vi "hostCommander.vi"() -> ()   [LabVIEW 2014]
uses:
  <vilib>/Platform/TimedLoop/XDataNode/timing_clust.ctl
  <vilib>/Platform/TimedLoop/XDataNode/nitl_modes.ctl
  <vilib>/Platform/TimedLoop/XDataNode/wakeup.ctl
  <vilib>/dex/Stream Element Allocation Mode.ctl
  <vilib>/platform/TimedLoop/XDataNode/XDataNode.xnode
  <resource>/objmgr/ni.dex.rc
  <vilib>/Platform/TimedLoop/XDataNode/XDNodeRunTimeDep.lvlib
  <vilib>/Analysis/NI_AALBase.lvlib
  <vilib>/Analysis/1siggen.llb/Riffle Array (I32).vi
panel:
  in  "Path":path
  in  "allowCorrection 2":bool
  out "Tab Control":enum32{"Host Commander"}(tab)
  out "rightReward":dbl format="%.2f"
  out "leftReward":dbl format="%.2f"
  out "rightLick":dbl format="%.2f"
  out "leftLick":dbl format="%.2f"
  out "reward#":i32=500
  in  "tickRate":u32=1
  in  "displayLength":dbl=10.0
  out "CurTrial#":u16
  out "Digital Waveform Graph":digitalwaveform(graph)
  out "stateMissed":bool
  out "VSmissed":bool
  out "VSbusy":bool=TRUE caption="VS"
  out "stateBusy":bool=TRUE caption="State"
  in  "FileName":string="debug"
  in  "Save data":bool=TRUE
  in  "Tab Control _2":T1(tab)
  in  "trialKey":i32[](array[numeric])
  in  "left":dbl=0.5 format="%.2f"
  in  "right":dbl=0.5 format="%.2f"
  in  "Initializeation Screen":dbl
  in  "Repeat":dbl
  in  "Interleave":bool
  in  "Randominze":bool
  in  "Blank":bool
  in  "Timing":sgl[](array[numeric])=[0.1, 0.2, 0.4, 0.6, 0.8, 1.0]
  in  "Orientation":sgl[](array[numeric])=[0.1, 0.2, 0.4, 0.6, 0.8, 1.0]
  in  "TF":sgl[](array[numeric])=[0.1, 0.2, 0.4, 0.6, 0.8, 1.0]
  in  "VS type":string="LR_FullFiledGrating"
  in  "SF":sgl[](array[numeric])=[0.04, 0.08, 0.16, 0.32, 0.45]
  in  "rtFIFOsize":u32=50
  in  "rtFIFOtimeout":u32
  in  "rtFIFOdataPool":u32=20
  in  "stateMachineCycle_uS":i64=500
  in  "minDelay":i32=2000000
  in  "maxDelay":i32=2000000
  in  "autoAllowCorrection":bool
  in  "allowCorrection":bool
  in  "autoDelay":bool
  in  "vsFilterPeriod_uS":i32=500 format="%#1.6f"
  in  "lickThreshold_V":fxp<+/-,16,5>=1.0 format="%#.4f"
  in  "vsThreshold_V":fxp<+/-,16,5>=2.0 format="%#.4f"
  in  "audioThreshold_V":fxp<+/-,16,5>=2.2998046875 format="%.4f"
  in  "audioFilterPeriod_uS":i32=500 format="%#1.6f"
  in  "audioOffState_V":fxp<+/-,16,5> format="%#.4f"
  in  "manualShock":bool
  in  "manualWaterRight":bool
  in  "manualWaterLeft":bool
  in  "lickReward":bool
  in  "allowPunish":bool
  in  "beh type":string="LeftRight"
  in  "toneReward":bool
  in  "rwdrefPeriod_uS":u32=1000000
  in  "rewardPeriod_uS":u32=3000000
  in  "waterOn_uS":u32=35000
  in  "timeout_uS":u32
  in  "shockOn_uS":u32
  in  "delay_uS":u32
  out "current state":u16(ring) items=["idle", "vs before", "vs", "vs after", "delay", "tone before", "tone", "tone after", "cycle end", "reward", "reward refractory", "punish", "punish refractory", "timeout", "exit"]
  out "case2":i32
  out "case1":i32
  in  "forceLeftTrial":bool
  in  "forceRightTrial":bool
  in  "forceCorrTrial":bool
  in  "autoCorrTrial":bool
  in  "autoTimeout":bool
  in  "autoStop":bool
  in  "autoStopAtReward#":i32=250
  in  "updateEveryTrial#":u16=10
  in  "maxTimeout":i32=8000000
  out "newStartTrial#":i32
  out "newStartReward#":i32
  out "contNoRewardAccum":i32
  out "contNoReward":i32
  out "contReward":i32
  out "curPerformance":dbl format="%.2f"
  out "overallPerformance":dbl format="%.2f"
  in  "waterPunish":bool
  out "Error 1":string
  out "Error 2":string
  out "Originating IP":string="192.168.137.2"
  out "Incoming data":string="TrlDone 1.000 "
  out "stream counter":u32
  out "Is Connected":bool
  out "Available Elements for Writing":i32
  in  "stream writer buffer size":i32=500
  in  "IP_VS":string="192.168.137.3"
  in  "IP_RT":string="192.168.137.2"
  in  "port_remote":u16=9091
  in  "IP_host":string="192.168.137.1"
  in  "port_local":u16=9090
  in  "IP_broadcast":string="192.168.137.255"
  out "INFO":string="Stop 1.000 "
  out "stop - local":bool=TRUE
  in  "Notes":string="14-4"
  in  "Abort":bool caption="run-stop"
  in  "run-stop":bool
  out "dispTimeout":bool
  out "saveTimeout":bool
  out "CurTrial# (remote)":u16
  in  "totalTrial#":u16=600
  out "CurTime":i32
  in  "ITI_ms":dbl=2000.0
  out "CurTime (sec)":i32
  in  "FilePath":string="D:\\BehData\\"
  # "busy"
  # "missed"
  # "min"
  # "sec"
  # "trialProbability"
  # "Errors for debugging"
types:
  T1 = enum32{"Visual Stimuli", "State Machine", "Behavior", "Network", "Notes"}
  T2 = enum16{"open", "replace", "create", "open or create", "replace or create", "replace or create with confirmation"}
  T3 = enum16{"big-endian, network order", "native, host order", "little-endian"}
  T4 = typedef "XDNodeRunTimeDep.lvlib/timing_clust.ctl" = cluster{"Expected End [f-1]":u64, "Actual End [f-1]":u64, "Finished Late? [f-1]":bool, "Expected End [i-1]":u64, "Actual End [i-1]":u64, "Finished Late? [i-1]":bool, "Expected Start [i]":u64, "Actual Start [i]":u64, "Expected Start [f]":u64, "Actual Start [f]":u64, "Source Name":string, "Structure Name":string, "Period":i64, "Deadline":i64, "Offset":i64, "Start":i64, "Priority":i32, "Timeout":i32, "Mode":T5, "Wakeup Reason":T6, "Error":errorcluster, "Source Type":string, "Secondary Source Type":string, "Global End Time":u64, "Global Start Time":u64, "Frame Duration":u64, "Iteration Duration":u64, "Assigned CPU":i32, "I/O Scan Engine Mode":u32}
  T5 = typedef "XDNodeRunTimeDep.lvlib/nitl_modes.ctl" = enum32{"No Change", "Process missed periods, maintain original phase", "Discard missed periods, maintain original phase", "Process missed periods, ignore original phase", "Discard missed periods, ignore original phase"}
  T6 = typedef "XDNodeRunTimeDep.lvlib/wakeup.ctl" = enum32{"Normal", "Aborted", "Asynchronous wakeup", "Timing source error", "Timed loop error", "Timeout"}
  T7 = typedef "Stream Element Allocation Mode.ctl" = u32
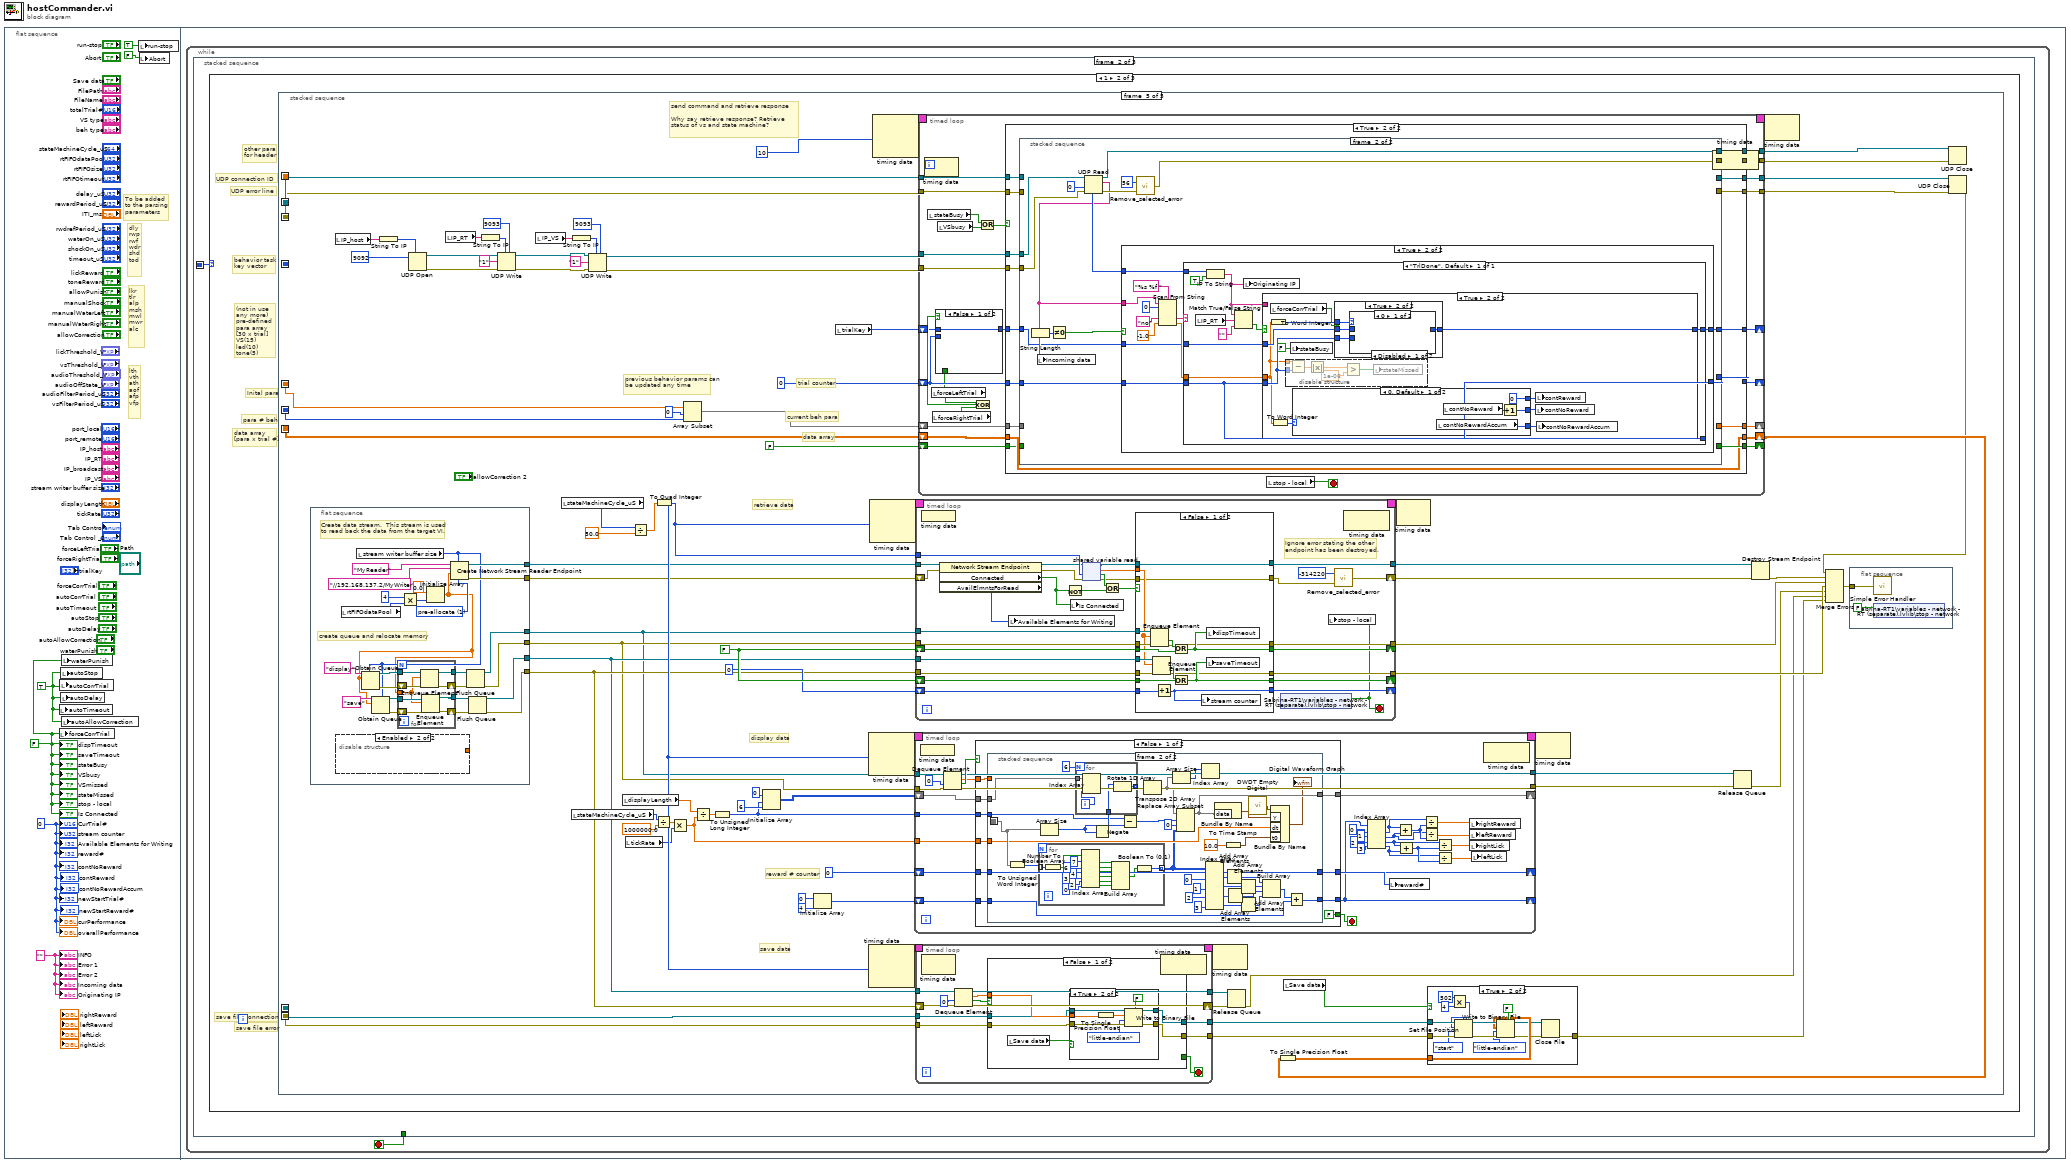
[diagram p0: block diagram]
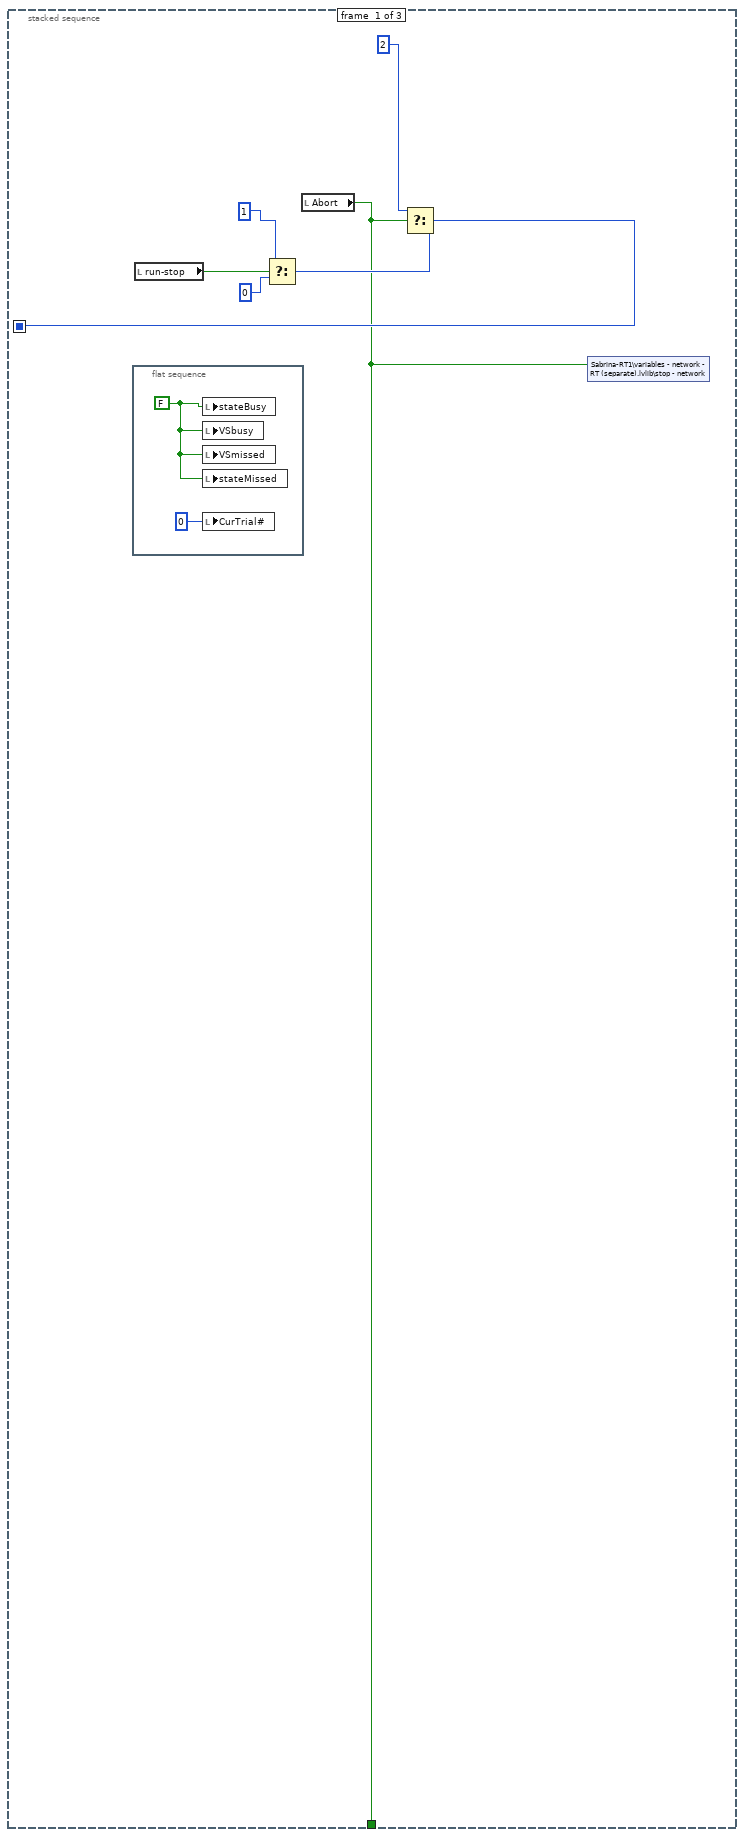
[diagram p2: hidden frame]
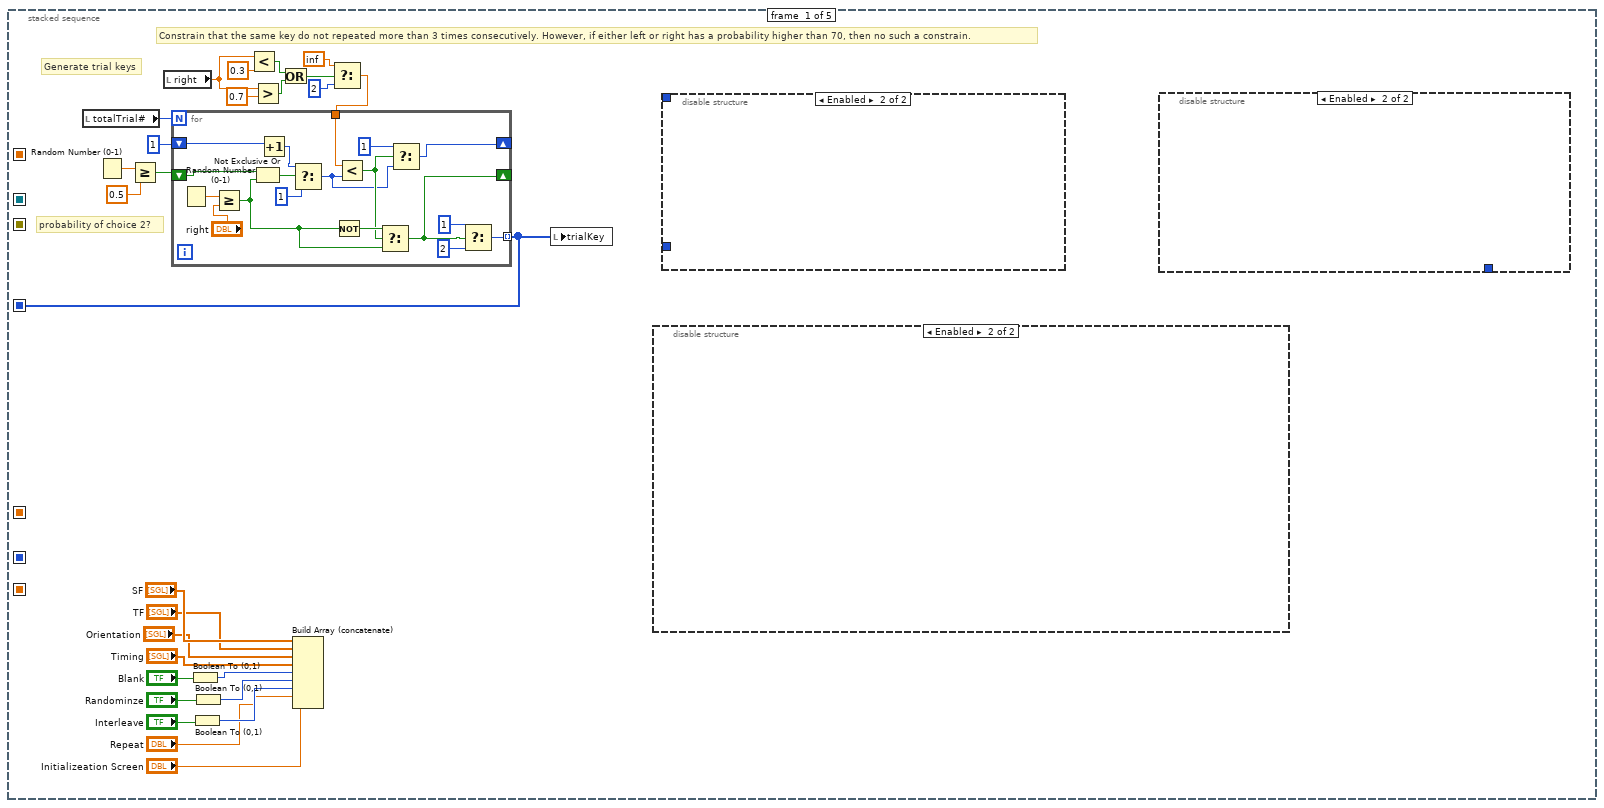
[diagram p4: hidden frame]
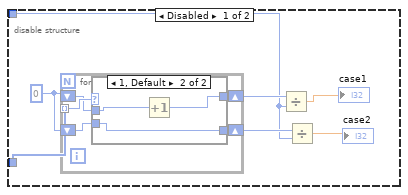
[diagram p5: hidden frame]
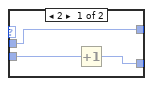
[diagram p6: hidden frame]
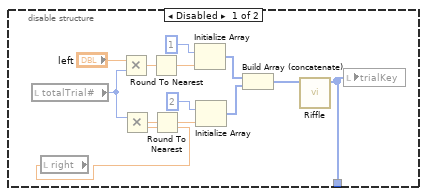
[diagram p7: hidden frame]
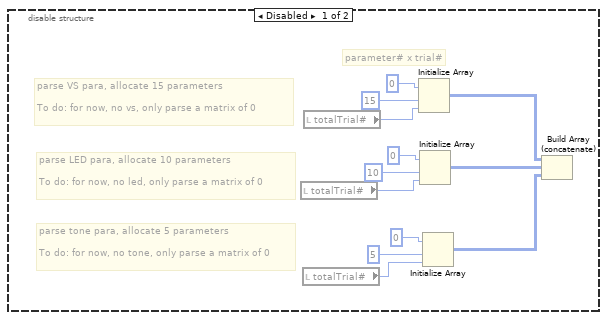
[diagram p8: hidden frame]
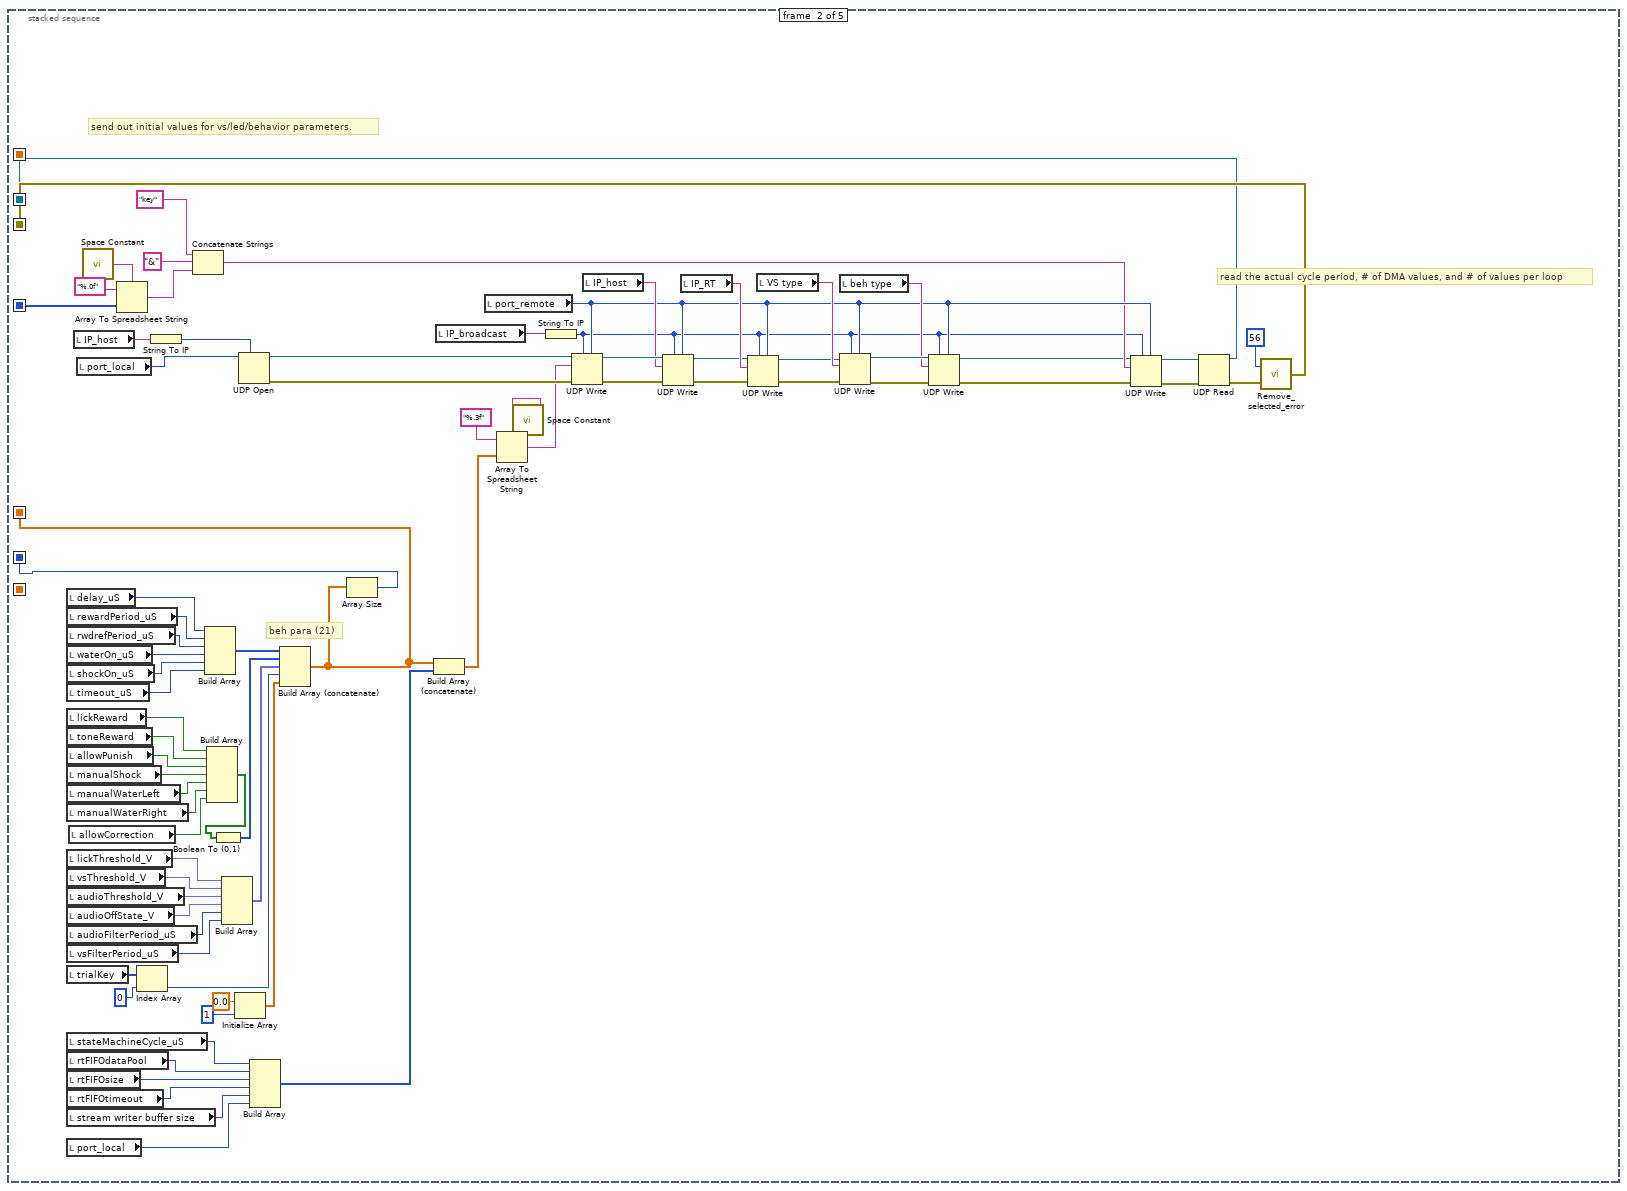
[diagram p9: hidden frame]
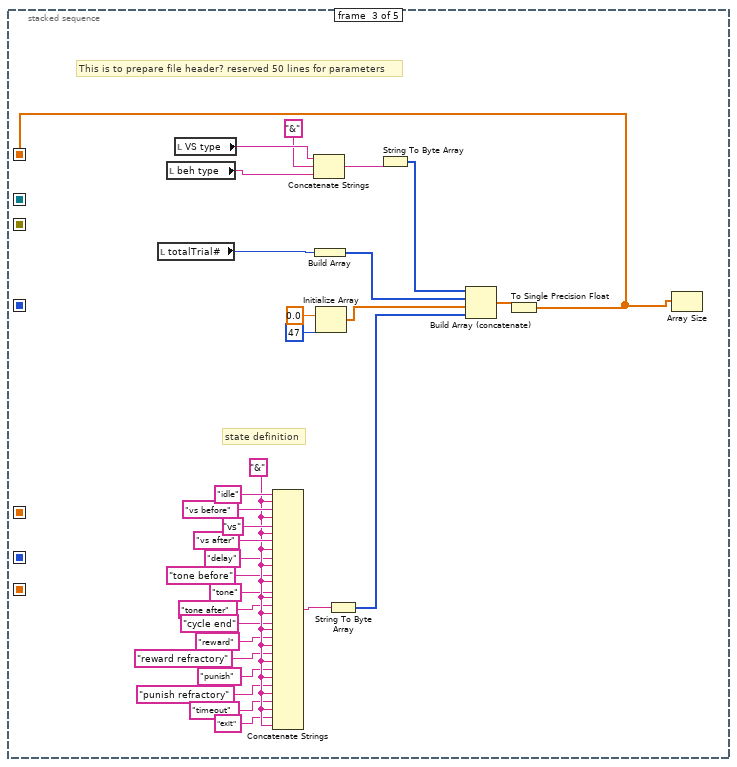
[diagram p10: hidden frame]
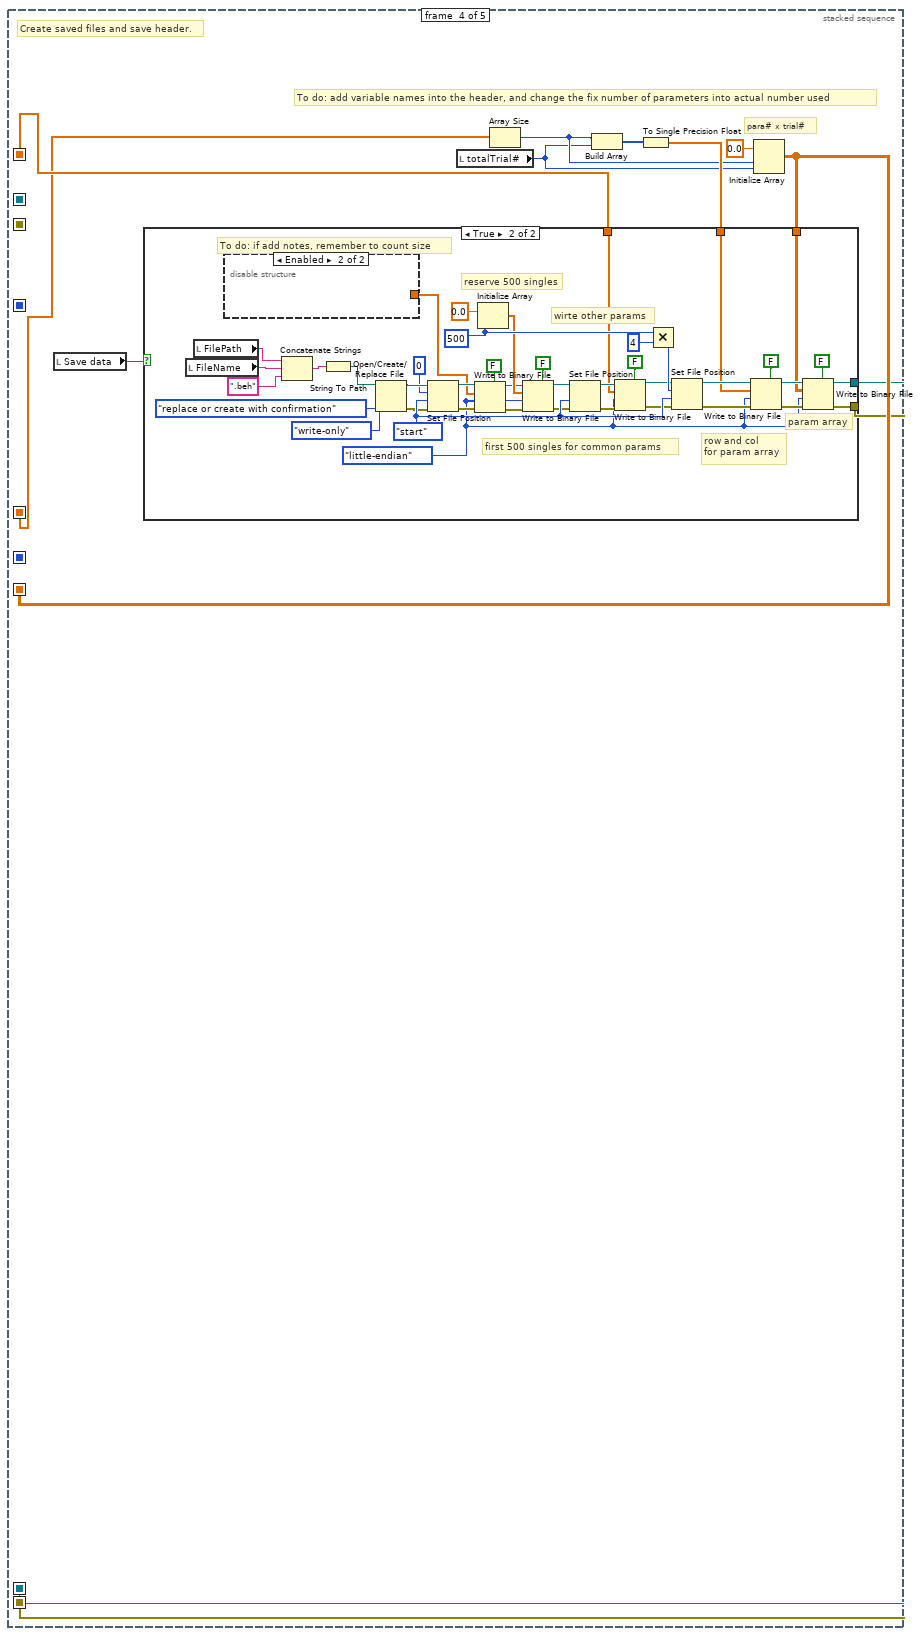
[diagram p11: hidden frame]
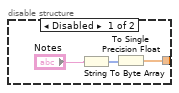
[diagram p13: hidden frame]
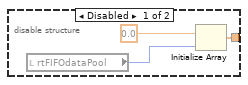
[diagram p14: hidden frame]
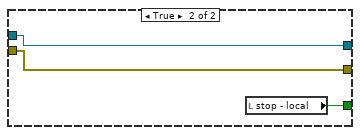
[diagram p16: hidden frame]
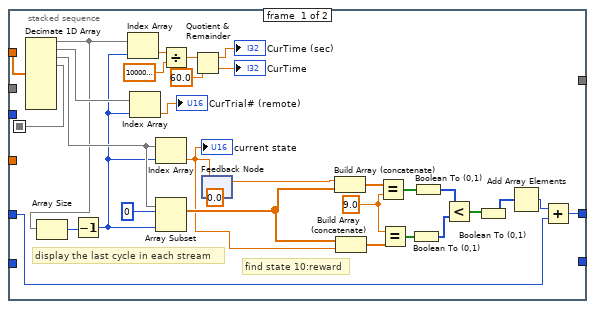
[diagram p17: hidden frame]
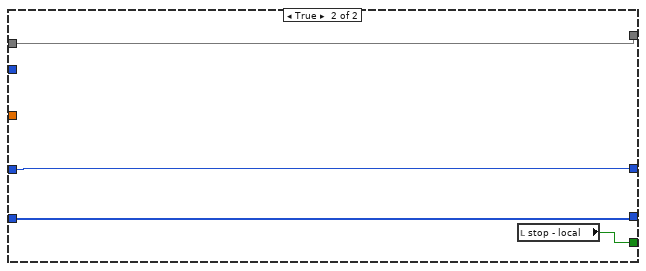
[diagram p18: hidden frame]
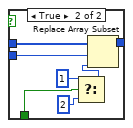
[diagram p20: hidden frame]
diagram:
  n1 = flat-sequence {
    frame #0 {
      w2 = TRUE
      w4 = ""
      w3 = 0
      w1 = FALSE
      # "To be added\nto the parsing\nparameters"
      # "lth\nvth\nath\naof\nafp\nvfp"
      # "dly\nrwp\nrwf\nwdr\nshd\ntod"
      # "lkr\ntlr\nalp\nmsh\nmwl\nmwr\nalc"
      n2 = local write "autoTimeout"(w2) -> ()
      n3 = local write "forceCorrTrial"(w1) -> ()
      n4 = local write "autoCorrTrial"(w2) -> ()
      n5 = local write "autoDelay"(w2) -> ()
      n6 = local write "autoStop"(w2) -> ()
      n7 = local write "waterPunish"(w1) -> ()
      n8 = local write "autoAllowCorrection"(w2) -> ()
      n9 = local write "run-stop"(TRUE) -> ()
      n10 = local write "Abort"(FALSE) -> ()
      "dispTimeout" <- w1
      "saveTimeout" <- w1
      "stateBusy" <- w1
      "VSbusy" <- w1
      "VSmissed" <- w1
      "stateMissed" <- w1
      "CurTrial#" <- w3
      "stop - local" <- w1
      "INFO" <- w4
      "Error 2" <- w4
      "Error 1" <- w4
      "Available Elements for Writing" <- w3
      "Is Connected" <- w1
      "stream counter" <- w3
      "Incoming data" <- w4
      "Originating IP" <- w4
      "reward#" <- w3
      "contNoReward" <- w3
      "contReward" <- w3
      "contNoRewardAccum" <- w3
      "newStartTrial#" <- w3
      "newStartReward#" <- w3
      "curPerformance" <- w3
      "overallPerformance" <- w3
    }
    frame #1 {
      n11 = while {
        stop <- w7 stop-if-true
        n12 = stacked-sequence {
          seq-local: [w9 _ _] -> [_ w17 _]
          tunnel: [w8 _ _] -> w7
          frame #0 {
            n13 = flat-sequence {
              frame #0 {
                w16 = FALSE
                n14 = local write "stateBusy"(w16) -> ()
                n15 = local write "VSbusy"(w16) -> ()
                n16 = local write "VSmissed"(w16) -> ()
                n17 = local write "stateMissed"(w16) -> ()
                n18 = local write "CurTrial#"(0) -> ()
              }
            }
            n19 = local read "run-stop"() -> (w11:bool)
            n20 = Select(t=u8 1, s=w11, f=u8 0) -> (s? t:f=w10:u8)
            n21 = local read "Abort"() -> (w8:bool)
            n22 = Select(t=u8 2, s=w8, f=w10) -> (s? t:f=w9:u8)
            n23 = shared-variable "Sabrina-RT1\\variables - network - RT (separate).lvlib\\stop - network"(w8) -> ()  [unwired: 1 in, 1 out]
          }
          frame #1 {
            n24 = case shown="1" w17 {
              frame 0, Default {
              }
              frame 1 {
                # "behavior task\nkey vector"
                # "para # beh"
                # "save file error"
                # "save file connection"
                # "data array\n[para x trial #]"
                # "other para\nfor header"
                # "UDP error line"
                # "UDP connection ID"
                # "Inital para"
                # "(not in use any more) pre-defined \npara array\n[30 x trial]\nVS(15)\nled(10)\ntone(5)"
                n25 = stacked-sequence {
                  seq-local: [_ w166 _ _ _] -> [_ _ _ _ w342]
                  seq-local: [_ w165 _ _ _] -> [_ _ _ _ w343]
                  seq-local: [_ w125 _ _ _] -> [_ _ _ w215 w291]
                  seq-local: [w18 _ _ _ _] -> [_ w121 _ _ _]
                  seq-local: [_ _ w183 _ _] -> [_ _ _ w219 _]
                  seq-local: [_ _ _ w218 _] -> [_ _ _ _ w336]
                  seq-local: [_ _ _ w217 _] -> [_ _ _ _ w316]
                  seq-local: [_ _ _ w216 _] -> [_ _ _ _ w317]
                  seq-local: [_ w134 _ _ _] -> [_ _ _ _ w297]
                  frame #0 {
                    # "probability of choice 2?"
                    # "Constrain that the same key do not repeated more than 3 times consecutively. However, if either left or right has a probability higher than 70, then no such a constrain."
                    # "Generate trial keys"
                    n26 = local read "totalTrial#"() -> (w19:u16)
                    n27 = Random Number (0-1)() -> (number: 0 to 1=w32:dbl)
                    n28 = Greater Or Equal?(x=w32, y=0.5) -> (x >= y?=w30:bool)
                    n29 = local read "right"() -> (w26:dbl)
                    n30 = Boolean To (0,1)(Boolean="Blank") -> (0, 1=w39:i16)
                    n31 = Boolean To (0,1)(Boolean="Interleave") -> (0, 1=w34:i16)
                    n32 = Boolean To (0,1)(Boolean="Randominze") -> (0, 1=w38:i16)
                    n33 = Less?(x=w26, y=0.3) -> (x < y?=w23:bool)
                    n34 = Greater?(x=w26, y=0.7) -> (0:w22:bool)
                    n35 = Or(x=w23, y=w22) -> (x .or. y?=w21:bool)
                    n36 = Build Array (concatenate)("SF", "TF", "Orientation", "Timing", w39, w38, w34, "Repeat", "Initializeation Screen") -> ()  [unwired: 1 out]
                    n37 = Select(t=inf, s=w21, f=2) -> (s? t:f=w20:dbl)
                    n38 = for {
                      N: w19 -> [_]
                      shift-right: [w79] -> _
                      shift-left: w30 -> [w92]
                      shift-right: [w77] -> _
                      shift-left: 1 -> [w90]
                      tunnel: w20 -> [w80]
                      tunnel: [w78] -> w18 mode=indexing
                      n39 = Random Number (0-1)() -> (number: 0 to 1=w93:dbl)
                      n40 = Greater Or Equal?(x=w93, y="right") -> (x >= y?=w83:bool)
                      n41 = Not Exclusive Or(1:w83, 2:w92) -> (0:w91:bool)
                      n42 = Increment(x=w90) -> (x+1=w87:i32)
                      n43 = Select(t=w87, s=w91, f=1) -> (s? t:f=w81:i32)
                      n44 = Not(x=w83) -> (.not. x?=w84:bool)
                      n45 = Less?(x=w80, y=w81) -> (x < y?=w82:bool)
                      n46 = Select(t=w84, s=w82, f=w83) -> (s? t:f=w79:bool)
                      n47 = Select(t=1, s=w82, f=w81) -> (s? t:f=w77:i32)
                      n48 = Select(t=1, s=w79, f=2) -> (s? t:f=w78:i32)
                    }
                    n49 = local write "trialKey"(w18) -> ()
                    n50 = disable-structure shown="Enabled" {
                      frame Disabled {
                        # "parameter# x trial#"
                        # "parse tone para, allocate 5 parameters \n\nTo do: for now, no tone, only parse a matrix of 0"
                        # "parse LED para, allocate 10 parameters \n\nTo do: for now, no led, only parse a matrix of 0"
                        # "parse VS para, allocate 15 parameters \n\nTo do: for now, no vs, only parse a matrix of 0"
                        n51 = local read "totalTrial#"() -> (w99:u16)
                        n52 = local read "totalTrial#"() -> (w98:u16)
                        n53 = local read "totalTrial#"() -> (w100:u16)
                        n54 = Initialize Array(0, 15, w100) -> (w103:i32[][])
                        n55 = Initialize Array(0, 10, w99) -> (w102:i32[][])
                        n56 = Initialize Array(0, 5, w98) -> (w101:i32[][])
                        n57 = Build Array (concatenate)(w103, w102, w101) -> ()  [unwired: 1 out]
                      }
                      frame Enabled {
                      }
                    }
                    n58 = disable-structure shown="Enabled" {
                      disable-tunnel: _ -> [w51 _]
                      disable-tunnel: _ -> [w45 _]
                      frame Disabled {
                        w50 = 0
                        n59 = for {
                          tunnel: w51 -> [w56] mode=indexing
                          shift-right: [w54] -> w47
                          shift-left: w50 -> [w55]
                          shift-right: [w52] -> w49
                          shift-left: w50 -> [w53]
                          n60 = case shown="1, Default" w56 {
                            tunnel: w55 -> [w59 w60]
                            tunnel: [w58 w60] -> w54
                            tunnel: w53 -> [w57 w62]
                            tunnel: [w57 w61] -> w52
                            frame 2 {
                              n61 = Increment(x=w59) -> (x+1=w58:i32)
                            }
                            frame 1, Default {
                              n62 = Increment(x=w62) -> (x+1=w61:i32)
                            }
                          }
                        }
                        n63 = Divide(x=w49, y=w45) -> (x/y=→"case1":dbl)
                        n64 = Divide(x=w47, y=w45) -> (x/y=→"case2":dbl)
                      }
                      frame Enabled {
                      }
                    }
                    n65 = disable-structure shown="Enabled" {
                      disable-tunnel: [w64 _] -> _
                      frame Disabled {
                        n66 = local read "totalTrial#"() -> (w68:u16)
                        n67 = local read "right"() -> (w63:dbl)
                        n68 = Multiply(x="left", y=w68) -> (x*y=w74:dbl)
                        n69 = Multiply(x=w68, y=w63) -> (x*y=w69:dbl)
                        n70 = Round To Nearest(number=w74) -> (nearest integer value=w72:dbl)
                        n71 = Round To Nearest(number=w69) -> (nearest integer value=w71:dbl)
                        n72 = Initialize Array(1, w72) -> (w67:i32[])
                        n73 = Initialize Array(2, w71) -> (w66:i32[])
                        n74 = Build Array (concatenate)(w67, w66) -> (w65:i32[])
                        n75 = call-poly <vilib>:"Riffle.vi"("X"=w65) -> ("Riffled {X}"=w64:i32[])  [unwired: 8 in, 2 out]
                        n76 = local write "trialKey"(w64) -> ()
                      }
                      frame Enabled {
                      }
                    }
                  }
                  frame #1 {
                    # "beh para (21)"
                    # "read the actual cycle period, # of DMA values, and # of values per loop"
                    # "send out initial values for vs/led/behavior parameters."
                    n77 = local read "delay_uS"() -> (w162:u32)
                    n78 = local read "rewardPeriod_uS"() -> (w161:u32)
                    n79 = local read "rwdrefPeriod_uS"() -> (w160:u32)
                    n80 = local read "waterOn_uS"() -> (w159:u32)
                    n81 = local read "shockOn_uS"() -> (w158:u32)
                    n82 = local read "timeout_uS"() -> (w157:u32)
                    n83 = local read "lickReward"() -> (w156:bool)
                    n84 = local read "toneReward"() -> (w155:bool)
                    n85 = local read "allowPunish"() -> (w154:bool)
                    n86 = local read "manualShock"() -> (w153:bool)
                    n87 = local read "manualWaterLeft"() -> (w152:bool)
                    n88 = local read "manualWaterRight"() -> (w151:bool)
                    n89 = local read "lickThreshold_V"() -> (w150:fxp<+/-,16,5>)
                    n90 = local read "vsThreshold_V"() -> (w149:fxp<+/-,16,5>)
                    n91 = local read "audioThreshold_V"() -> (w148:fxp<+/-,16,5>)
                    n92 = local read "audioOffState_V"() -> (w145:fxp<+/-,16,5>)
                    n93 = local read "audioFilterPeriod_uS"() -> (w147:i32)
                    n94 = local read "vsFilterPeriod_uS"() -> (w146:i32)
                    n95 = local read "trialKey"() -> (w110:i32[])
                    n96 = local read "stateMachineCycle_uS"() -> (w144:i64)
                    n97 = local read "rtFIFOdataPool"() -> (w142:u32)
                    n98 = local read "rtFIFOsize"() -> (w141:u32)
                    n99 = local read "rtFIFOtimeout"() -> (w143:u32)
                    n100 = local read "stream writer buffer size"() -> (w140:i32)
                    n101 = local read "port_local"() -> (w133:u16)
                    n102 = local read "allowCorrection"() -> (w106:bool)
                    n103 = local read "IP_host"() -> (w179:string)
                    n104 = local read "port_local"() -> (w178:u16)
                    n105 = call <vilib>:"Space Constant.vi"() -> ("String"=w115:string)
                    n106 = Array To Spreadsheet String ("beh para")(delimiter (Tab)=w115, array=w121, 3:"%.0f" ("format string")) -> (spreadsheet string=w117:string)
                    n107 = Index Array(array=w110, index=0) -> (element=w107:i32)
                    n108 = String To IP(1:w179) -> (0:w111:u32)
                    n109 = Concatenate Strings("key", "&", w117) -> (w116:string)
                    n110 = Build Array(w162, w161, w160, w159, w158, w157) -> (w139:u32[])
                    n111 = Build Array(w156, w155, w154, w153, w152, w151, w106) -> (w127:bool[])
                    n112 = Boolean To (0,1)(Boolean=w127) -> (0, 1=w126:i16[])
                    n113 = Build Array(w150, w149, w148, w145, w147, w146) -> (w138:fxp<+/-,43,32>[])
                    n114 = Initialize Array(sgl 0.0, 1) -> (w108:sgl[])
                    n115 = UDP Open(7:w111, 11:w178) -> (port=w176:refnum<k16>, 0:w177:errorcluster)  [unwired: 3 in, 1 out]
                    n116 = Build Array(w144, w142, w141, w143, w140, w133) -> (w137:i64[])
                    n117 = Build Array (concatenate)(w139, w126, w138, w107, w108) -> (w125:sgl[])
                    n118 = Array Size(array=w125) -> (size(s)=w134:i32)
                    n119 = Build Array (concatenate)(w125, w137) -> (w167:sgl[])
                    n120 = local read "IP_broadcast"() -> (w180:string)
                    n121 = local read "port_remote"() -> (w118:u16)
                    n122 = call <vilib>:"Space Constant.vi"() -> ("String"=w169:string)
                    n123 = Array To Spreadsheet String ("beh para")(delimiter (Tab)=w169, array=w167, 3:"%.3f" ("format string")) -> (spreadsheet string=w168:string)
                    n124 = String To IP(1:w180) -> (0:w112:u32)
                    n125 = UDP Write(address=w112, port or service name=w118, connection ID=w176, data in=w168, 8:w177) -> (error out=w175:errorcluster, 3:w132:refnum<k16>)  [unwired: 1 in]
                    n126 = local read "IP_host"() -> (w131:string)
                    n127 = UDP Write(address=w112, port or service name=w118, connection ID=w132, data in=w131) -> (3:w129:refnum<k16>)  [unwired: 2 in, 1 out]
                    n128 = local read "IP_RT"() -> (w130:string)
                    n129 = UDP Write(address=w112, port or service name=w118, connection ID=w129, data in=w130) -> (3:w128:refnum<k16>)  [unwired: 2 in, 1 out]
                    n130 = local read "VS type"() -> (w174:string)
                    n131 = local read "beh type"() -> (w171:string)
                    n132 = UDP Write(address=w112, port or service name=w118, connection ID=w128, data in=w174, 8:w175) -> (error out=w173:errorcluster, 3:w172:refnum<k16>)  [unwired: 1 in]
                    n133 = UDP Write(address=w112, port or service name=w118, connection ID=w172, data in=w171, 8:w173) -> (error out=w113:errorcluster, 3:w114:refnum<k16>)  [unwired: 1 in]
                    n134 = UDP Write(address=w112, port or service name=w118, connection ID=w114, data in=w116, 8:w113) -> (error out=w124:errorcluster, 3:w123:refnum<k16>)  [unwired: 1 in]
                    n135 = UDP Read(connection ID=w123, 8:w124) -> (error out=w164:errorcluster, 3:w165:refnum<k16>)  [unwired: 2 in, 3 out]
                    n136 = call "Remove_selected_error.vi"("error in (no error)"=w164, "errorCode"=56) -> ("error out"=w166:errorcluster)
                  }
                  frame #2 {
                    w195 = "&" ("string")
                    # "state definition"
                    # "This is to prepare file header? reserved 50 lines for parameters"
                    n137 = local read "totalTrial#"() -> (w203:u16)
                    n138 = local read "beh type"() -> (w181:string)
                    n139 = local read "VS type"() -> (w198:string)
                    n140 = Concatenate Strings("idle", w195, "vs before", w195, "vs", w195, "vs after", w195, "delay", w195, "tone before", w195, "tone", w195, "tone after", w195, "cycle end", w195, "reward", w195, "reward refractory", w195, "punish", w195, "punish refractory", w195, "timeout", w195, "exit", w195) -> (w208:string)
                    n141 = Concatenate Strings(w198, "&" ("string"), w181) -> (w197:string)
                    n142 = Build Array(w203) -> (w202:u16[])
                    n143 = Initialize Array(sgl 0.0 ("element"), 47 ("dimension size")) -> (w201:sgl[])
                    n144 = String To Byte Array(string=w208) -> (unsigned byte array=w200:u8[])
                    n145 = String To Byte Array(string=w197) -> (unsigned byte array=w196:u8[])
                    n146 = Build Array (concatenate)(w196, w202, w201, w200) -> (w199:sgl[])
                    n147 = To Single Precision Float(number=w199) -> (single precision float=w183:sgl[])
                    n148 = Array Size(array=w183) -> ()  [unwired: 1 out]
                  }
                  frame #3 {
                    # "To do: add variable names into the header, and change the fix number of parameters into actual number used"
                    # "para# x trial#"
                    # "Create saved files and save header."
                    n149 = local read "Save data"() -> (w221:bool)
                    n150 = local read "totalTrial#"() -> (w211:u16)
                    n151 = Array Size(array=w215) -> (size(s)=w212:i32)
                    n152 = Build Array(w212, w211) -> (w214:i32[])
                    n153 = To Single Precision Float(number=w214) -> (single precision float=w213:sgl[])
                    n154 = Initialize Array(sgl 0.0 ("element"), w212, w211) -> (w218:sgl[][])
                    n155 = case shown="True" w221 {
                      tunnel: w213 -> [_ w238]
                      tunnel: w219 -> [_ w222]
                      tunnel: w218 -> [_ w237]
                      tunnel: [_ w235] -> w216
                      tunnel: [_ w236] -> w217
                      frame False {
                      }
                      frame True {
                        w256 = 500 ("dimension size")
                        w229 = T3."little-endian" ("byte order (0:big-endian, network order)")
                        w257 = enum16{"start", "end", "current"}."start" ("from (0:start)")
                        # "To do: if add notes, remember to count size"
                        # "param array"
                        # "row and col\nfor param array"
                        # "first 500 singles for common params"
                        # "reserve 500 singles"
                        # "wirte other params"
                        n156 = local read "FileName"() -> (w224:string)
                        n157 = local read "FilePath"() -> (w227:string)
                        n158 = disable-structure shown="Enabled" {
                          disable-tunnel: [w264 _] -> w228
                          frame Disabled {
                            n159 = String To Byte Array(string="Notes") -> (unsigned byte array=w265:u8[])
                            n160 = To Single Precision Float(number=w265) -> (single precision float=w264:sgl[])
                          }
                          frame Enabled {
                          }
                        }
                        n161 = Concatenate Strings(w227, w224, ".beh" ("string")) -> (w226:string)
                        n162 = String To Path(string=w226) -> (path=w225:path)
                        n163 = Open/Create/Replace File(file path (use dialog)=w225, operation (0:open)=T2."replace or create with confirmation", access (0:read/write)=enum16{"read/write", "read-only", "write-only"}."write-only") -> (refnum out=w242:refnum<file>, error out=w243:errorcluster)  [unwired: 3 in, 1 out]
                        n164 = Set File Position(offset (in bytes) (0)=i64 0, refnum=w242, from (0:start)=w257, error in=w243) -> (refnum out=w233:refnum<file>, error out=w231:errorcluster)
                        n165 = Write to Binary File(file (use dialog)=w233, data=w228, error in=w231, 5:FALSE ("prepend array or string size? (T)"), 9:w229) -> (refnum out=w232:refnum<file>, error out=w230:errorcluster)  [unwired: 1 in, 1 out]
                        n166 = Initialize Array(sgl 0.0 ("element"), w256) -> (w246:sgl[])
                        n167 = Write to Binary File(file (use dialog)=w232, data=w246, error in=w230, 5:FALSE ("prepend array or string size? (T)"), 9:w229) -> (refnum out=w248:refnum<file>, error out=w249:errorcluster)  [unwired: 1 in, 1 out]
                        n168 = Set File Position(refnum=w248, from (0:start)=w257, error in=w249) -> (refnum out=w250:refnum<file>, error out=w251:errorcluster)  [unwired: 1 in]
                        n169 = Write to Binary File(file (use dialog)=w250, data=w222, error in=w251, 5:FALSE ("prepend array or string size? (T)"), 9:w229) -> (refnum out=w252:refnum<file>, error out=w253:errorcluster)  [unwired: 1 in, 1 out]
                        n170 = Multiply(x=w256, y=4) -> (x*y=w254:i32)
                        n171 = Set File Position(offset (in bytes) (0)=w254, refnum=w252, from (0:start)=w257, error in=w253) -> (refnum out=w259:refnum<file>, error out=w260:errorcluster)
                        n172 = Write to Binary File(file (use dialog)=w259, data=w238, error in=w260, 5:FALSE ("prepend array or string size? (T)"), 9:w229) -> (refnum out=w261:refnum<file>, error out=w262:errorcluster)  [unwired: 1 in, 1 out]
                        n173 = Write to Binary File(file (use dialog)=w261, data=w237, error in=w262, 5:FALSE ("prepend array or string size? (T)"), 9:w229) -> (refnum out=w235:refnum<file>, error out=w236:errorcluster)  [unwired: 1 in, 1 out]
                      }
                    }
                  }
                  frame #4 {
                    w348 = FALSE
                    # "reward # counter"
                    # "save data"
                    # "data array"
                    # "current beh para"
                    # "trial counter"
                    # "previous behavior params can be updated any time"
                    # "display data"
                    # "retrieve data"
                    # "send command and retrieve response\n\nWhy say retrieve response? Retrieve\nstatus of vs and state machine?"
                    n174 = flat-sequence {
                      tunnel: [w375] -> w303
                      tunnel: [w374] -> w302
                      tunnel: [w363] -> w301
                      tunnel: [w362] -> w300
                      tunnel: [w361] -> w299
                      tunnel: [w360] -> w298
                      frame #0 {
                        w377 = T7 1 items=["allocate as needed", "pre-allocate"] ("element allocation mode")
                        # "create queue and relocate memory"
                        # "Create data stream.  This stream is used\nto read back the data from the target VI."
                        n175 = disable-structure shown="Enabled" {
                          disable-tunnel: [w380 _] -> _
                          frame Disabled {
                            n176 = local read "rtFIFOdataPool"() -> (w381:u32)
                            n177 = Initialize Array(sgl 0.0, w381) -> (w380:sgl[])
                          }
                          frame Enabled {
                          }
                        }
                        n178 = local read "rtFIFOdataPool"() -> (w356:u32)
                        n179 = local read "stream writer buffer size"() -> (w359:i32)
                        n180 = Multiply(x=4, y=w356) -> (x*y=w355:u32)
                        n181 = Initialize Array(sgl 0.0, w355) -> (w358:sgl[])
                        n182 = Obtain Queue(max queue size (-1, unlimited)=w359, name (unnamed)="display", element data type=w358) -> (queue out=w366:refnum<queue>, error out=w367:errorcluster)  [unwired: 2 in, 1 out]
                        n183 = Obtain Queue(max queue size (-1, unlimited)=w359, name (unnamed)="save", element data type=w358) -> (queue out=w368:refnum<queue>, error out=w369:errorcluster)  [unwired: 2 in, 1 out]
                        n184 = for {
                          N: w359 -> [_]
                          tunnel: w366 -> [w391]
                          tunnel: [w390] -> w372
                          shift-right: [w388] -> w373
                          shift-left: w367 -> [w389]
                          shift-right: [w384] -> w371
                          shift-left: w369 -> [w385]
                          tunnel: w368 -> [w387]
                          tunnel: [w386] -> w370
                          tunnel: w358 -> [w383]
                          n185 = Enqueue Element(queue=w391, element=w383, error in (no error)=w389) -> (queue out=w390:refnum<queue>, error out=w388:errorcluster)  [unwired: 1 in, 1 out]
                          n186 = Enqueue Element(queue=w387, element=w383, error in (no error)=w385) -> (queue out=w386:refnum<queue>, error out=w384:errorcluster)  [unwired: 1 in, 1 out]
                        }
                        n187 = Create Network Stream Reader Endpoint(6:w377, 7:w359, 9:w358, 10:"//192.168.137.2/MyWriter" ("reader name"), 11:"MyReader" ("reader name")) -> (0:w375:errorcluster, 3:w374:refnum<k21>)  [unwired: 2 in]
                        n188 = Flush Queue(queue=w372, error in (no error)=w373) -> (queue out=w360:refnum<queue>, error out=w361:errorcluster)  [unwired: 1 out]
                        n189 = Flush Queue(queue=w370, error in (no error)=w371) -> (queue out=w362:refnum<queue>, error out=w363:errorcluster)  [unwired: 1 out]
                      }
                    }
                    n190 = local read "IP_host"() -> (w286:string)
                    n191 = String To IP(1:w286) -> (0:w285:u32)
                    n192 = UDP Open(7:w285, 11:9092) -> (port=w280:refnum<k16>, 0:w281:errorcluster)  [unwired: 3 in, 1 out]
                    n193 = local read "IP_RT"() -> (w279:string)
                    n194 = String To IP(1:w279) -> (0:w278:u32)
                    n195 = UDP Write(address=w278, port or service name=u16 9093, connection ID=w280, data in="1", 8:w281) -> (error out=w270:errorcluster, 3:w271:refnum<k16>)  [unwired: 1 in]
                    n196 = local read "IP_VS"() -> (w272:string)
                    n197 = local read "stateMachineCycle_uS"() -> (w351:i64)
                    n198 = local read "stateMachineCycle_uS"() -> (w330:i64)
                    n199 = String To IP(1:w272) -> (0:w273:u32)
                    n200 = UDP Write(address=w273, port or service name=u16 9093, connection ID=w271, data in="1", 8:w270) -> (error out=w268:errorcluster, 3:w269:refnum<k16>)  [unwired: 1 in]
                    n201 = local read "displayLength"() -> (w324:dbl)
                    n202 = local read "tickRate"() -> (w295:u32)
                    n203 = Divide(x=w351, y=sgl 50.0) -> (x/y=w350:sgl)
                    n204 = To Quad Integer(1:w350) -> (0:w304:i64)
                    n205 = Divide(x=w330, y=1000000.0) -> (x/y=w296:dbl)
                    n206 = Multiply(x=w296, y=w295) -> (x*y=w294:dbl)
                    n207 = Array Subset(array=w291, index=0, length=w297) -> (w341:sgl[])
                    n208 = Divide(x=w324, y=w294) -> (x/y=w327:dbl)
                    n209 = To Unsigned Long Integer(number=w327) -> (unsigned 32bit integer=w325:u32)
                    n210 = Initialize Array(u8 0, w325, 6 ("dimension size")) -> (w326:u8[][])
                    n211 = Initialize Array(u32 0, u32 4) -> (w288:u32[])
                    n212 = local read "trialKey"() -> (w267:i32[])
                    n213 = node-c288(w304) -> (w323:T4)  [unwired: 2 in]
                    n214 = node-c288(w304) -> (w321:T4)  [unwired: 2 in]
                    n215 = node-c288(w304) -> (w354:T4)  [unwired: 2 in]
                    n216 = node-c288(10) -> (w345:T4)  [unwired: 2 in]
                    n217 = timed-loop {
                      tunnel: w298 -> [w460]
                      tunnel: w299 -> [w459]
                      shift-right: [w431] -> _
                      shift-left: u32 0 -> [w448]
                      shift-right: [w454] -> _
                      shift-left: w326 -> [w456]
                      tunnel: w325 -> [w455]
                      timing: w323 -> [_]
                      timing-out: [_] -> w322
                      tunnel: [w451] -> w313
                      tunnel: [w450] -> w312
                      tunnel: w294 -> [w449]
                      shift-right: [w442] -> _
                      shift-left: w288 -> [w447]
                      stop <- w453 stop-if-true
                      n218 = node-c288() -> ()  [unwired: 1 in]
                      n219 = Dequeue Element(queue=w460, timeout in ms (-1)=0, error in (no error)=w459) -> (queue out=w451:refnum<queue>, element=w457:sgl[], timed out?=w458:bool, error out=w450:errorcluster)
                      n220 = case shown="False" w458 {
                        tunnel: w457 -> [w472 _]
                        tunnel: w448 -> [w471 w561]
                        tunnel: [w470 w561] -> w431
                        tunnel: w456 -> [w469 w562]
                        tunnel: w455 -> [w468 _]
                        tunnel: [w467 w562] -> w454
                        tunnel: [FALSE w563] -> w453
                        tunnel: w449 -> [w465 _]
                        tunnel: w447 -> [w464 w560]
                        tunnel: [w463 w560] -> w442
                        frame False {
                          n221 = stacked-sequence {
                            seq-local: [w474 _] -> [_ w531]
                            tunnel: w472 -> [w503 _]
                            tunnel: w471 -> [w488 _]
                            tunnel: [w493 _] -> w470
                            tunnel: w469 -> [_ w530]
                            tunnel: w468 -> [_ w522]
                            tunnel: [_ w525] -> w467
                            tunnel: w465 -> [_ w523]
                            tunnel: w464 -> [_ w505]
                            tunnel: [_ w504] -> w463
                            frame #0 {
                              w482 = sgl 9.0
                              # "display the last cycle in each stream"
                              # "find state 10:reward"
                              n222 = Decimate 1D Array(w503) -> (w489:sgl[], w491:sgl[], w490:sgl[], w474:sgl[])  [unwired: 5 out]
                              n223 = Array Size(array=w489) -> (size(s)=w487:i32)
                              n224 = Decrement(x=w487) -> (x-1=w486:i32)
                              n225 = Index Array(array=w489, index=w486) -> (element=w494:sgl)
                              n226 = Index Array(array=w491, index=w486) -> (element=→"CurTrial# (remote)":sgl)
                              n227 = Index Array(array=w490, index=w486) -> (element=w484:sgl)
                              "current state" <- w484
                              n228 = Array Subset(array=w490, index=0, length=w486) -> (w485:sgl[])
                              n229 = Divide(x=w494, y=sgl 1000000.0) -> (x/y=w496:sgl)
                              n230 = Quotient & Remainder(x=w496, y=sgl 60.0) -> (x-y*floor(x/y)=→"CurTime (sec)":sgl, floor(x/y)=→"CurTime":sgl)
                              n231 = feedback #1(sgl 0.0) -> (w499:sgl)
                              n232 = feedback-in #1(w484) -> ()
                              n233 = Build Array (concatenate)(w499, w485) -> (w483:sgl[])
                              n234 = Build Array (concatenate)(w485, w484) -> (w481:sgl[])
                              n235 = Equal?(x=w483, y=w482) -> (x = y?=w479:bool[])
                              n236 = Equal?(x=w482, y=w481) -> (x = y?=w478:bool[])
                              n237 = Boolean To (0,1)(Boolean=w478) -> (0, 1=w476:i16[])
                              n238 = Boolean To (0,1)(Boolean=w479) -> (0, 1=w477:i16[])
                              n239 = Less?(x=w477, y=w476) -> (x < y?=w480:bool[])
                              n240 = Boolean To (0,1)(Boolean=w480) -> (0, 1=w501:i16[])
                              n241 = Add Array Elements(numeric array=w501) -> (sum=w502:i16)
                              n242 = Add(x=w502, y=w488) -> (x+y=w493:u32)
                            }
                            frame #1 {
                              n243 = To Unsigned Word Integer(number=w531) -> (unsigned 16bit integer=w532:u16[])
                              n244 = for {
                                tunnel: w532 -> [w559] mode=indexing
                                tunnel: [w546] -> w514 mode=indexing
                                n245 = Number To Boolean Array(number=w559) -> (Boolean array=w558:bool[])
                                n246 = Index Array(array=w558, index #1=7, index #2=6, index #3=4, index #4=3, index #5=2, index #6=0) -> (element #1=w557:bool, element #2=w556:bool, element #3=w555:bool, element #4=w554:bool, element #5=w553:bool, element #6=w545:bool)
                                n247 = Build Array(w557, w556, w555, w554, w553, w545) -> (w547:bool[])
                                n248 = Boolean To (0,1)(Boolean=w547) -> (0, 1=w546:i16[])
                              }
                              n249 = Array Size(array=w531) -> (size(s)=w538:i32)
                              n250 = Negate(x=w538) -> (-x=w536:i32)
                              n251 = for {
                                N: 6 -> [_]
                                tunnel: w530 -> [w543]
                                tunnel: w536 -> [w540]
                                tunnel: [w539] -> w537 mode=indexing
                                i -> [w542]
                                n252 = Index Array(array=w543, index (col)=w542) -> (element=w541:u8[])  [unwired: 1 in]
                                n253 = Rotate 1D Array(1:w541, 2:w540) -> (0:w539:u8[])
                              }
                              n254 = Subtract(x=w522, y=w538) -> (x-y=w533:u32)
                              n255 = Transpose 2D Array(2D array=w537) -> (transposed array=w520:u8[][])
                              n256 = Array Size(array=w520) -> (size(s)=w521:i32[])
                              n257 = Replace Array Subset(array=w520, new element=w514, index (row)=w533, index (col)=0 ("disabled index (col)")) -> (w525:u8[][])
                              n258 = Index Array(array=w521) -> ()  [unwired: 1 in, 1 out]
                              n259 = Index Array(array=w514, index (col) #1=0, index (col) #2=1, index (col) #3=2, index (col) #4=3) -> (element #1=w515:i16[], element #2=w513:i16[], element #3=w512:i16[], element #4=w511:i16[])  [unwired: 4 in]
                              n260 = Bundle By Name ("Build Digital Data")("data"=w525) -> (w527:digitaldata)  [unwired: 1 in]
                              n261 = To Time Stamp(1:10.0 ("number")) -> (0:w529:timestamp)
                              n262 = Add Array Elements(numeric array=w515) -> (sum=w510:i16)
                              n263 = Add Array Elements(numeric array=w512) -> (sum=w509:i16)
                              n264 = Add Array Elements(numeric array=w513) -> (sum=w507:i16)
                              n265 = Add Array Elements(numeric array=w511) -> (sum=w508:i16)
                              n266 = call <vilib>:"DWDT Empty Digital.vi"() -> ("digital waveform out"=w526:digitalwaveform)  [unwired: 5 in]
                              n267 = Build Array(w510, w507, w509, w508) -> (w506:i16[])
                              n268 = Bundle By Name ("Build Waveform")(cluster=w526, "Y"=w527, "dt"=w523, "t0"=w529) -> (→"Digital Waveform Graph":digitalwaveform)
                              n269 = Add(x=w506, y=w505) -> (x+y=w504:u32[])
                            }
                          }
                        }
                        frame True {
                          n270 = local read "stop - local"() -> (w563:bool)
                        }
                      }
                      n271 = Index Array(array=w442, index #1=0, index #2=1, index #3=2, index #4=3) -> (element #1=w439:u32, element #2=w440:u32, element #3=w437:u32, element #4=w436:u32)
                      n272 = local write "reward#"(w448) -> ()
                      n273 = Add(x=w439, y=w440) -> (x+y=w441:u32)
                      n274 = Add(x=w437, y=w436) -> (x+y=w438:u32)
                      n275 = Divide(x=w439, y=w441) -> (x/y=w432:dbl)
                      n276 = Divide(x=w440, y=w441) -> (x/y=w433:dbl)
                      n277 = Divide(x=w437, y=w438) -> (x/y=w435:dbl)
                      n278 = Divide(x=w436, y=w438) -> (x/y=w434:dbl)
                      n279 = local write "rightReward"(w432) -> ()
                      n280 = local write "leftReward"(w433) -> ()
                      n281 = local write "rightLick"(w435) -> ()
                      n282 = local write "leftLick"(w434) -> ()
                      n283 = node-c288() -> ()  [unwired: 1 in, 1 out]
                    }
                    n284 = timed-loop {
                      timing: w321 -> [_]
                      timing-out: [_] -> w320
                      tunnel: w300 -> [w404]
                      tunnel: [w400] -> w319
                      shift-right: [w399] -> w318
                      shift-left: w301 -> [w403]
                      tunnel: w317 -> [w398]
                      tunnel: w316 -> [w397]
                      tunnel: [w396] -> w315
                      tunnel: [w395] -> w314
                      stop <- w394 stop-if-true
                      n285 = node-c288() -> ()  [unwired: 1 in, 1 out]
                      n286 = Dequeue Element(queue=w404, timeout in ms (-1)=0, error in (no error)=w403) -> (queue out=w400:refnum<queue>, element=w401:sgl[], timed out?=w402:bool, error out=w399:errorcluster)
                      n287 = case shown="False" w402 {
                        tunnel: w401 -> [w410 _]
                        tunnel: w398 -> [w409 w424]
                        tunnel: w397 -> [w408 w423]
                        tunnel: [w407 w424] -> w396
                        tunnel: [w406 w423] -> w395
                        tunnel: [_ w422] -> w394
                        frame False {
                          n288 = local read "Save data"() -> (w411:bool)
                          n289 = case shown="True" w411 {
                            tunnel: w409 -> [w412 w421]
                            tunnel: w408 -> [w413 w420]
                            tunnel: w410 -> [_ w415]
                            tunnel: [w413 w417] -> w406
                            tunnel: [w412 w416] -> w407
                            frame False {
                            }
                            frame True {
                              n290 = To Single Precision Float(number=w415) -> (single precision float=w414:sgl[])
                              n291 = Write to Binary File(file (use dialog)=w421, data=w414, error in=w420, 5:FALSE ("prepend array or string size? (T)"), 9:T3."little-endian" ("byte order (0:big-endian, network order)")) -> (refnum out=w416:refnum<file>, error out=w417:errorcluster)  [unwired: 1 in, 1 out]
                            }
                          }
                        }
                        frame True {
                          n292 = local read "stop - local"() -> (w422:bool)
                        }
                      }
                      n293 = node-c288() -> ()  [unwired: 1 in, 1 out]
                    }
                    n294 = timed-loop {
                      timing: w354 -> [_]
                      timing-out: [_] -> w353
                      tunnel: w304 -> [w1100]
                      tunnel: [w1118] -> w349
                      tunnel: w302 -> [w1117]
                      tunnel: w298 -> [w1116]
                      tunnel: w299 -> [w1115]
                      tunnel: w300 -> [w1114]
                      tunnel: w301 -> [w1113]
                      shift-right: [w1111] -> _
                      shift-left: w348 -> [w1112]
                      shift-right: [w1109] -> _
                      shift-left: w348 -> [w1110]
                      tunnel: [w1108] -> w306
                      tunnel: [w1107] -> w309
                      shift-right: [w1105] -> _
                      shift-left: u32 0 -> [w1106]
                      shift-right: [w1097] -> w346
                      shift-left: w303 -> [w1098]
                      stop <- w1094 stop-if-true
                      # "Ignore error stating the other\nendpoint has been destroyed."
                      n295 = node-c288() -> ()  [unwired: 1 in]
                      n296 = property class="Network Stream Endpoint"(reference=w1117, error in=w1098) -> (reference out=w1096:refnum<k21>, error out=w1101:errorcluster, "Connected"=w1121:bool, "AvailElmntsForRead"=w1122:i32)
                      n297 = local write "Available Elements for Writing"(w1122) -> ()
                      n298 = Not(x=w1121) -> (.not. x?=w1120:bool)
                      n299 = local write "Is Connected"(w1121) -> ()
                      n300 = shared-variable-read(w1096, w1101, w1100) -> (w1103:refnum<k21>, w1099:errorcluster, w1104:bool, w1102:sgl[])
                      n301 = Or(x=w1104, y=w1120) -> (x .or. y?=w1119:bool)
                      n302 = case shown="False" w1119 {
                        tunnel: w1103 -> [w1135 w1146]
                        tunnel: [w1135 w1146] -> w1118
                        tunnel: w1116 -> [w1139 _]
                        tunnel: w1115 -> [w1137 w1143]
                        tunnel: w1114 -> [w1138 _]
                        tunnel: w1113 -> [w1136 w1142]
                        tunnel: w1112 -> [w1133 w1145]
                        tunnel: [w1129 w1145] -> w1111
                        tunnel: w1110 -> [w1132 w1144]
                        tunnel: [w1131 w1144] -> w1109
                        tunnel: [w1128 w1143] -> w1108
                        tunnel: [w1127 w1142] -> w1107
                        tunnel: w1106 -> [w1126 w1141]
                        tunnel: [w1125 w1141] -> w1105
                        tunnel: w1102 -> [w1124 _]
                        tunnel: [w1123 w1140] -> w1095
                        tunnel: w1099 -> [w1123 w1140]
                        frame False {
                          n303 = Enqueue Element(queue=w1139, element=w1124, error in (no error)=w1137) -> (timed out?=w1134:bool, error out=w1128:errorcluster)  [unwired: 1 in, 1 out]
                          n304 = Enqueue Element(queue=w1138, element=w1124, error in (no error)=w1136) -> (timed out?=w1130:bool, error out=w1127:errorcluster)  [unwired: 1 in, 1 out]
                          n305 = Increment(x=w1126) -> (x+1=w1125:u32)
                          n306 = Or(x=w1134, y=w1133) -> (x .or. y?=w1129:bool)
                          n307 = Or(x=w1130, y=w1132) -> (x .or. y?=w1131:bool)
                          n308 = local write "stream counter"(w1125) -> ()
                          n309 = local write "saveTimeout"(w1131) -> ()
                          n310 = local write "dispTimeout"(w1129) -> ()
                        }
                        frame True {
                        }
                      }
                      n311 = shared-variable "Sabrina-RT1\\variables - network - RT (separate).lvlib\\stop - network"() -> (w1094:bool)  [unwired: 1 in, 1 out]
                      n312 = local write "stop - local"(w1094) -> ()
                      n313 = call "Remove_selected_error.vi"("error in (no error)"=w1095, "errorCode"=-314220) -> ("error out"=w1097:errorcluster)
                      n314 = node-c288() -> ()  [unwired: 1 in, 1 out]
                    }
                    n315 = timed-loop {
                      timing: w345 -> [_]
                      timing-out: [_] -> w344
                      tunnel: w343 -> [w605]
                      tunnel: w342 -> [w604]
                      shift-right: [w602] -> _
                      shift-left: w341 -> [w603]
                      tunnel: [w601] -> w340
                      tunnel: [w600] -> w339
                      shift-right: [w599] -> _
                      shift-left: 0 ("index") -> [w589]
                      shift-right: [w597] -> _
                      shift-left: FALSE -> [w598]
                      shift-right: [w595] -> w333
                      shift-left: w336 -> [w596]
                      tunnel: w269 -> [w593]
                      tunnel: w268 -> [w592]
                      tunnel: [w591] -> w283
                      tunnel: [w590] -> w282
                      shift-right: [w583] -> _
                      shift-left: w267 -> [w584]
                      stop <- w594 stop-if-true
                      n316 = node-c288() -> ()  [unwired: 1 in, 1 out]
                      n317 = local read "stateBusy"() -> (w608:bool)
                      n318 = local read "forceLeftTrial"() -> (w586:bool)
                      n319 = local read "forceRightTrial"() -> (w588:bool)
                      n320 = local read "VSbusy"() -> (w607:bool)
                      n321 = Exclusive Or(1:w588, 2:w586) -> (0:w587:bool)
                      n322 = case shown="False" w587 {
                        tunnel: w589 -> [_ w611]
                        tunnel: w586 -> [_ w613]
                        tunnel: [w609 w612] -> w585
                        tunnel: w584 -> [w609 w610]
                        frame False {
                        }
                        frame True {
                          n323 = Select(t=1 ("index"), s=w613, f=2 ("index")) -> (s? t:f=w616:i32)
                          n324 = Replace Array Subset(array=w610, new element=w616, index=w611) -> (w612:i32[])
                        }
                      }
                      n325 = Or(x=w608, y=w607) -> (x .or. y?=w606:bool)
                      n326 = case shown="True" w606 {
                        tunnel: w605 -> [w630 w892]
                        tunnel: w604 -> [w623 w891]
                        tunnel: w603 -> [w633 w890]
                        tunnel: [w622 w889] -> w602
                        tunnel: [w629 w888] -> w601
                        tunnel: [w624 w887] -> w600
                        tunnel: w589 -> [w620 w886]
                        tunnel: [w635 w885] -> w599
                        tunnel: w598 -> [w634 w882]
                        tunnel: [w621 w884] -> w597
                        tunnel: w596 -> [w632 w883]
                        tunnel: [w631 w883] -> w595
                        tunnel: [w619 w878] -> w591
                        tunnel: [w618 w879] -> w590
                        tunnel: w593 -> [w619 w881]
                        tunnel: w592 -> [w618 w880]
                        tunnel: w585 -> [w617 w877]
                        tunnel: [w617 w876] -> w583
                        frame False {
                          n327 = stacked-sequence {
                            seq-local: [_ w764 _] -> [_ _ w869]
                            tunnel: w620 -> [_ w759 w871]
                            tunnel: [_ _ w870] -> w635
                            tunnel: w634 -> [_ w803 _]
                            tunnel: w633 -> [_ w801 _]
                            tunnel: w632 -> [_ w761 _]
                            tunnel: [_ w795 _] -> w631
                            tunnel: [_ w793 _] -> w626
                            tunnel: [_ w769 _] -> w622
                            tunnel: [_ w764 _] -> w621
                            tunnel: w617 -> [_ w757 _]
                            frame #0 {
                              n328 = local read "CurTrial#"() -> (w638:u16)
                              n329 = local read "autoTimeout"() -> (w648:bool)
                              n330 = case shown="True" w648 {
                                frame False {
                                }
                                frame True {
                                n331 = local read "curPerformance"() -> (w713:dbl)
                                n332 = local read "overallPerformance"() -> (w715:dbl)
                                n333 = local read "reward#"() -> (w716:i32)
                                n334 = Less?(x=w713, y=0.7) -> (x < y?=w718:bool)
                                n335 = Less?(x=w716, y=10 ("index")) -> (x < y?=w722:bool)
                                n336 = Less?(x=w715, y=0.3) -> (x < y?=w724:bool)
                                n337 = Or(x=w722, y=w724) -> (x .or. y?=w719:bool)
                                n338 = Not(x=w719) -> (.not. x?=w717:bool)
                                n339 = And(x=w717, y=w718) -> (x .and. y?=w720:bool)
                                n340 = case shown="True" w720 {
                                tunnel: [w728 w730] -> w721
                                frame False {
                                n341 = local read "timeout_uS"() -> (w728:u32)
                                }
                                frame True {
                                n342 = local read "CurTrial#"() -> (w729:u16)
                                n343 = Quotient & Remainder(x=w729, y="updateEveryTrial#") -> (x-y*floor(x/y)=w738:u16)  [unwired: 1 out]
                                n344 = Equal?(x=0.0, y=w738) -> (x = y?=w737:bool)
                                n345 = local read "timeout_uS"() -> (w734:u32)
                                n346 = Add(x=1000000, y=w734) -> (x+y=w735:u32)
                                n347 = Select(t=w735, s=w737, f=w734) -> (s? t:f=w732:u32)
                                n348 = Less?(x=w732, y="maxTimeout") -> (x < y?=w733:bool)
                                n349 = Select(t=w732, s=w733, f="maxTimeout") -> (s? t:f=w730:u32)
                                }
                                }
                                n350 = Select(t=0, s=w719, f=w721) -> (s? t:f=w726:u32)
                                n351 = local write "timeout_uS"(w726) -> ()
                                }
                              }
                              n352 = local read "reward#"() -> (w639:i32)
                              n353 = local read "autoCorrTrial"() -> (w649:bool)
                              n354 = Divide(x=w639, y=w638) -> (x/y=w637:dbl)
                              n355 = local write "overallPerformance"(w637) -> ()
                              n356 = case shown="True" w649 {
                                frame False {
                                }
                                frame True {
                                n357 = local read "overallPerformance"() -> (w741:dbl)
                                n358 = local read "rightReward"() -> (w750:dbl)
                                n359 = local read "leftReward"() -> (w742:dbl)
                                n360 = local read "reward#"() -> (w743:i32)
                                n361 = Greater Or Equal?(x=w743, y=10 ("index")) -> (x >= y?=w746:bool)
                                n362 = Max & Min(x=w750, y=w742) -> (max(x,y)=w754:dbl)  [unwired: 1 out]
                                n363 = Greater Or Equal?(x=w741, y=0.5) -> (x >= y?=w744:bool)
                                n364 = Less?(x=w754, y=0.55 ("number")) -> (x < y?=w747:bool)
                                n365 = And(x=w747, y=w744) -> (x .and. y?=w745:bool)
                                n366 = Select(t=FALSE, s=w745, f=w746) -> (s? t:f=w752:bool)
                                n367 = local write "forceCorrTrial"(w752) -> ()
                                }
                              }
                              n368 = local read "autoDelay"() -> (w636:bool)
                              n369 = case shown="True" w636 {
                                tunnel: [w650 w654] -> w640
                                frame False {
                                n370 = local read "overallPerformance"() -> (w650:dbl)
                                }
                                frame True {
                                n371 = local read "reward#"() -> (w651:i32)
                                n372 = Greater?(x=w651, y=u16 11) -> (0:w652:bool)
                                n373 = case shown="True" w652 {
                                tunnel: [w661 w669] -> w654
                                tunnel: w651 -> [w659 w662]
                                frame False {
                                n374 = Equal?(x=w659, y=u16 11) -> (x = y?=w658:bool)
                                n375 = local read "overallPerformance"() -> (w661:dbl)
                                n376 = Select(t="minDelay", s=w658, f=u32 0 ("delay_uS")) -> (s? t:f=w655:u32)
                                n377 = local write "delay_uS"(w655) -> ()
                                }
                                frame True {
                                n378 = local read "newStartReward#"() -> (w671:i32)
                                n379 = local read "newStartTrial#"() -> (w673:i32)
                                n380 = local read "contNoRewardAccum"() -> (w672:i32)
                                n381 = local read "CurTrial# (remote)"() -> (w663:u16)
                                n382 = Subtract(x=w662, y=w671) -> (x-y=w664:i32)
                                n383 = local read "contReward"() -> (w674:i32)
                                n384 = Subtract(x=w663, y=w673) -> (x-y=w667:i32)
                                n385 = Subtract(x=w667, y=w672) -> (x-y=w670:i32)
                                n386 = Less?(x=10 ("index"), y=w667) -> (x < y?=w666:bool)
                                n387 = Greater Or Equal?(x=w674, y=4) -> (x >= y?=w679:bool)
                                n388 = Divide(x=w664, y=w670) -> (x/y=w669:dbl)
                                n389 = Greater?(x=w662, y=14) -> (0:w678:bool)
                                n390 = And(x=w678, y=w679) -> (x .and. y?=w677:bool)
                                n391 = Greater?(x=w669, y=0.7 ("number")) -> (0:w665:bool)
                                n392 = Compound Arithmetic op=AND(w677, w666, w665) -> (w680:bool)
                                n393 = case shown="True" w680 {
                                tunnel: w663 -> [_ w687]
                                tunnel: w662 -> [_ w686]
                                frame False {
                                }
                                frame True {
                                w683 = 0
                                n394 = local read "delay_uS"() -> (w688:u32)
                                n395 = local write "newStartReward#"(w686) -> ()
                                n396 = local write "newStartTrial#"(w687) -> ()
                                n397 = Add(x=w688, y=200000.0 ("number")) -> (x+y=w682:dbl)
                                n398 = local write "contNoRewardAccum"(w683) -> ()
                                n399 = local write "contReward"(w683) -> ()
                                n400 = Max & Min(x="maxDelay", y=w682) -> (min(x,y)=w684:dbl)  [unwired: 1 out]
                                n401 = local write "delay_uS"(w684) -> ()
                                }
                                }
                                }
                                }
                                }
                              }
                              n402 = local read "autoAllowCorrection"() -> (w643:bool)
                              n403 = local read "contNoReward"() -> (w646:i32)
                              n404 = local read "autoStop"() -> (w647:bool)
                              n405 = case shown="True" w647 {
                                frame False {
                                }
                                frame True {
                                n406 = local read "overallPerformance"() -> (w703:dbl)
                                n407 = Multiply(x=0.9 ("y"), y="autoStopAtReward#") -> (x*y=w697:dbl)
                                n408 = Less?(x=w703, y=0.7) -> (x < y?=w700:bool)
                                n409 = local read "waterPunish"() -> (w701:bool)
                                n410 = And(x=w700, y=w701) -> (x .and. y?=w702:bool)
                                n411 = Select(t=w697, s=w702, f="autoStopAtReward#") -> (s? t:f=w707:dbl)
                                n412 = local read "contNoReward"() -> (w705:i32)
                                n413 = local read "reward#"() -> (w711:i32)
                                n414 = Greater Or Equal?(x=w711, y=w707) -> (x >= y?=w710:bool)
                                n415 = Greater?(x=w705, y=20 ("index")) -> (0:w704:bool)
                                n416 = Or(x=w710, y=w704) -> (x .or. y?=w709:bool)
                                n417 = case shown="True" w709 {
                                frame False {
                                }
                                frame True {
                                n418 = local write "run-stop"(FALSE) -> ()
                                }
                                }
                                }
                              }
                              n419 = Greater?(x=w646, y=5 ("index")) -> (0:w644:bool)
                              n420 = And(x=w644, y=w643) -> (x .and. y?=w642:bool)
                              n421 = case shown="False" w642 {
                                tunnel: [w690 TRUE] -> w641
                                frame False {
                                n422 = local read "reward#"() -> (w695:i32)
                                n423 = Greater Or Equal?(x=w695, y=10 ("index")) -> (x >= y?=w693:bool)
                                n424 = Select(t=FALSE, s=w693, f=TRUE) -> (s? t:f=w690:bool)
                                }
                                frame True {
                                }
                              }
                              n425 = local write "allowCorrection"(w641) -> ()
                              n426 = local write "curPerformance"(w640) -> ()
                            }
                            frame #1 {
                              # "beh para (20)"
                              n427 = local read "delay_uS"() -> (w791:u32)
                              n428 = local read "rewardPeriod_uS"() -> (w790:u32)
                              n429 = local read "rwdrefPeriod_uS"() -> (w789:u32)
                              n430 = local read "waterOn_uS"() -> (w788:u32)
                              n431 = local read "shockOn_uS"() -> (w787:u32)
                              n432 = local read "timeout_uS"() -> (w786:u32)
                              n433 = local read "lickReward"() -> (w785:bool)
                              n434 = local read "toneReward"() -> (w784:bool)
                              n435 = local read "allowPunish"() -> (w783:bool)
                              n436 = local read "manualShock"() -> (w782:bool)
                              n437 = local read "manualWaterLeft"() -> (w781:bool)
                              n438 = local read "manualWaterRight"() -> (w780:bool)
                              n439 = local read "lickThreshold_V"() -> (w779:fxp<+/-,16,5>)
                              n440 = local read "vsThreshold_V"() -> (w778:fxp<+/-,16,5>)
                              n441 = local read "audioThreshold_V"() -> (w777:fxp<+/-,16,5>)
                              n442 = local read "audioOffState_V"() -> (w774:fxp<+/-,16,5>)
                              n443 = local read "audioFilterPeriod_uS"() -> (w776:i32)
                              n444 = local read "vsFilterPeriod_uS"() -> (w775:i32)
                              n445 = local read "allowCorrection"() -> (w755:bool)
                              n446 = Index Array(array=w757, index=w759) -> (element=w760:i32)
                              n447 = Build Array(w791, w790, w789, w788, w787, w786) -> (w773:u32[])
                              n448 = Build Array(w785, w784, w783, w782, w781, w780, w755) -> (w766:bool[])
                              n449 = Boolean To (0,1)(Boolean=w766) -> (0, 1=w765:i16[])
                              n450 = Build Array(w779, w778, w777, w774, w776, w775) -> (w772:fxp<+/-,43,32>[])
                              n451 = Initialize Array(sgl 0.0, 1) -> (w756:sgl[])
                              n452 = Build Array (concatenate)(w773, w765, w772, w760, w756) -> (w769:sgl[])
                              n453 = Array Size(array=w769) -> (size(s)=w768:i32)
                              n454 = Subtract(x=w769, y=w801) -> (x-y=w800:sgl[])
                              n455 = Reshape Array(w769, w768, 1 ("dimension size")) -> (w796:sgl[][])
                              n456 = Absolute Value(x=w800) -> (abs(x)=w798:sgl[])
                              n457 = Less?(x=w798, y=1e-06) -> (x < y?=w797:bool[])
                              n458 = Replace Array Subset(array=w761, new element=w796, index (row)=0 ("dimension size"), index (col)=w759) -> (w795:sgl[][])
                              n459 = for {
                                N: 19 ("dimension size") -> [_]
                                tunnel: w797 -> [w840] mode=indexing
                                tunnel: w769 -> [w839] mode=indexing
                                shift-right: [w836] -> w794
                                shift-left: "" -> [w837]
                                i -> [w838]
                                n460 = case shown="False" w840 {
                                tunnel: w839 -> [_ w849]
                                tunnel: w838 -> [_ w843]
                                tunnel: w837 -> [w841 w847]
                                tunnel: [w841 w846] -> w836
                                frame True {
                                }
                                frame False {
                                n461 = case shown="3" w843 {
                                tunnel: ["dly" "rwp" "rwf" "wdr" "shd" "tod" "lkr" "tlr" "alp" "msh" "mwl" "mwr" "alc" "lth" "vth" "ath" "aof" "afp" _ _ _] -> w842
                                frame 0, Default {
                                }
                                frame 1 {
                                }
                                frame 2 {
                                }
                                frame 3 {
                                }
                                frame 4 {
                                }
                                frame 5 {
                                }
                                frame 6 {
                                }
                                frame 7 {
                                }
                                frame 8 {
                                }
                                frame 9 {
                                }
                                frame 10 {
                                }
                                frame 11 {
                                }
                                frame 12 {
                                }
                                frame 13 {
                                }
                                frame 14 {
                                }
                                frame 15 {
                                }
                                frame 16 {
                                }
                                frame 17 {
                                }
                                frame 18 {
                                (unwired) "vfp"
                                }
                                frame 19 {
                                }
                                frame 20 {
                                }
                                }
                                n462 = Format Value(format string="%.3f", value (0)=w849) -> (output string=w844:string)  [unwired: 1 in]
                                n463 = call <vilib>:"Space Constant.vi"() -> ("String"=w845:string)
                                n464 = Concatenate Strings(w847, w842, w845, w844, w845) -> (w846:string)
                                }
                                }
                              }
                              n465 = local read "VSmissed"() -> (w806:bool)
                              n466 = local read "stateMissed"() -> (w805:bool)
                              n467 = local read "CurTrial#"() -> (w809:u16)
                              n468 = local read "totalTrial#"() -> (w808:u16)
                              n469 = local read "run-stop"() -> (w804:bool)
                              n470 = Equal?(x=w809, y=w808) -> (x = y?=w807:bool)
                              n471 = Not(x=w804) -> (.not. x?=w802:bool)
                              n472 = Compound Arithmetic op=OR(w806, w805, w807) -> (w792:bool)
                              n473 = case shown="True" w792 {
                                frame False {
                                }
                                frame True {
                                n474 = local write "run-stop"(FALSE ("run-stop")) -> ()
                                }
                              }
                              n475 = Compound Arithmetic op=OR(w792, w802, w803) -> (w764:bool)
                              n476 = case shown="True" w764 {
                                tunnel: w794 -> [w813 _]
                                tunnel: [w812 w832] -> w793
                                tunnel: w760 -> [w810 _]
                                frame False {
                                n477 = flat-sequence {
                                tunnel: w813 -> [w814]
                                tunnel: [w814] -> w811
                                tunnel: [w828] -> w812
                                tunnel: w811 -> [w831]
                                tunnel: w810 -> [w825]
                                frame #0 {
                                n478 = disable-structure shown="Enabled" {
                                frame Disabled {
                                n479 = Random Number (0-1)() -> (number: 0 to 1=w817:dbl)
                                n480 = Multiply(x=w817, y=3000.0) -> (x*y=w819:dbl)
                                n481 = local read "ITI_ms"() -> (w815:dbl)
                                n482 = Add(x=w815, y=w819) -> (x+y=w818:dbl)
                                n483 = Wait (ms)(milliseconds to wait=w818) -> ()  [unwired: 1 out]
                                }
                                frame Enabled {
                                n484 = Random Number (0-1)() -> (number: 0 to 1=w822:dbl)
                                n485 = local read "ITI_ms"() -> (w820:dbl)
                                n486 = Multiply(x=w822, y=0) -> (x*y=w821:dbl)
                                n487 = Add(x=w820, y=w821) -> (x+y=w823:dbl)
                                n488 = Wait (ms)(milliseconds to wait=w823) -> ()  [unwired: 1 out]
                                }
                                }
                                }
                                frame #1 {
                                n489 = call <vilib>:"Space Constant.vi"() -> ("String"=w829:string)
                                n490 = Format Value(format string="%.3f", value (0)=w825) -> (output string=w826:string)  [unwired: 1 in]
                                n491 = Concatenate Strings(w831, "start" ("string"), w829, w826, w829) -> (w828:string)
                                }
                                }
                                }
                                frame True {
                                n492 = call <vilib>:"Space Constant.vi"() -> ("String"=w834:string)
                                n493 = Concatenate Strings("stop" ("string"), w834, "1.000" ("string"), w834) -> (w832:string)
                                n494 = call "generateTone.vi"() -> ()  [unwired: 12 in]
                                }
                              }
                            }
                            frame #2 {
                              n495 = case shown="False" w869 {
                                tunnel: w871 -> [w872 w875]
                                tunnel: [w872 w874] -> w870
                                frame True {
                                }
                                frame False {
                                w873 = TRUE
                                n496 = Increment(x=w875) -> (x+1=w874:i32)
                                n497 = local write "CurTrial#"(w874) -> ()
                                n498 = local write "stateBusy"(w873) -> ()
                                n499 = local write "VSbusy"(w873) -> ()
                                }
                              }
                            }
                          }
                          n500 = local write "INFO"(w626) -> ()
                          n501 = local read "IP_broadcast"() -> (w627:string)
                          n502 = local read "port_remote"() -> (w625:u16)
                          n503 = String To IP(1:w627) -> (0:w628:u32)
                          n504 = UDP Write(address=w628, port or service name=w625, connection ID=w630, data in=w626, 8:w623) -> (error out=w624:errorcluster, 3:w629:refnum<k16>)  [unwired: 1 in]
                        }
                        frame True {
                          n505 = stacked-sequence {
                            tunnel: w892 -> [w946 _]
                            tunnel: w891 -> [w945 _]
                            tunnel: w890 -> [w941 _]
                            tunnel: [w904 _] -> w889
                            tunnel: [w899 _] -> w888
                            tunnel: [w900 _] -> w887
                            tunnel: w886 -> [w897 w999]
                            tunnel: [_ w998] -> w885
                            tunnel: [w927 _] -> w884
                            tunnel: w882 -> [w901 _]
                            tunnel: w881 -> [_ w997]
                            tunnel: w880 -> [_ w996]
                            tunnel: [_ w995] -> w878
                            tunnel: [_ w994] -> w879
                            tunnel: w877 -> [w894 w992]
                            tunnel: [_ w991] -> w876
                            frame #0 {
                              # "triakKey is not used here, may be deleted"
                              # "beh para (21)"
                              n506 = local read "delay_uS"() -> (w926:u32)
                              n507 = local read "rewardPeriod_uS"() -> (w925:u32)
                              n508 = local read "rwdrefPeriod_uS"() -> (w924:u32)
                              n509 = local read "waterOn_uS"() -> (w923:u32)
                              n510 = local read "shockOn_uS"() -> (w922:u32)
                              n511 = local read "timeout_uS"() -> (w921:u32)
                              n512 = local read "lickReward"() -> (w920:bool)
                              n513 = local read "toneReward"() -> (w919:bool)
                              n514 = local read "allowPunish"() -> (w918:bool)
                              n515 = local read "manualShock"() -> (w917:bool)
                              n516 = local read "manualWaterLeft"() -> (w916:bool)
                              n517 = local read "manualWaterRight"() -> (w915:bool)
                              n518 = local read "lickThreshold_V"() -> (w914:fxp<+/-,16,5>)
                              n519 = local read "vsThreshold_V"() -> (w913:fxp<+/-,16,5>)
                              n520 = local read "audioThreshold_V"() -> (w912:fxp<+/-,16,5>)
                              n521 = local read "audioOffState_V"() -> (w909:fxp<+/-,16,5>)
                              n522 = local read "audioFilterPeriod_uS"() -> (w911:i32)
                              n523 = local read "vsFilterPeriod_uS"() -> (w910:i32)
                              n524 = local read "allowCorrection"() -> (w893:bool)
                              n525 = Index Array(array=w894, index=w897) -> (element=w896:i32)
                              n526 = Build Array(w926, w925, w924, w923, w922, w921) -> (w908:u32[])
                              n527 = Build Array(w920, w919, w918, w917, w916, w915, w893) -> (w903:bool[])
                              n528 = Boolean To (0,1)(Boolean=w903) -> (0, 1=w902:i16[])
                              n529 = Build Array(w914, w913, w912, w909, w911, w910) -> (w907:fxp<+/-,43,32>[])
                              n530 = Initialize Array(sgl 0.0, 1) -> (w898:sgl[])
                              n531 = Build Array (concatenate)(w908, w902, w907, w896, w898) -> (w904:sgl[])
                              n532 = Subtract(x=w904, y=w941) -> (x-y=w944:sgl[])
                              n533 = Absolute Value(x=w944) -> (abs(x)=w943:sgl[])
                              n534 = Less?(x=w943, y=1e-06) -> (x < y?=w940:bool[])
                              n535 = for {
                                N: 19 ("dimension size") -> [_]
                                tunnel: w940 -> [w949] mode=indexing
                                shift-right: [w950] -> w936
                                shift-left: "" -> [w951]
                                tunnel: w904 -> [w948] mode=indexing
                                i -> [w952]
                                n536 = case shown="False" w949 {
                                tunnel: w952 -> [w960 _]
                                tunnel: w951 -> [w956 w980]
                                tunnel: [w954 w980] -> w950
                                tunnel: w948 -> [w953 _]
                                frame False {
                                n537 = case shown="15" w960 {
                                tunnel: ["dly" "rwp" "rwf" "wdr" "shd" "tod" "lkr" "tlr" "alp" "msh" "mwl" "mwr" "alc" "lth" "vth" "ath" "aof" "afp" "vfp" _ _] -> w955
                                frame 0, Default {
                                }
                                frame 1 {
                                }
                                frame 2 {
                                }
                                frame 3 {
                                }
                                frame 4 {
                                }
                                frame 5 {
                                }
                                frame 6 {
                                }
                                frame 7 {
                                }
                                frame 8 {
                                }
                                frame 9 {
                                }
                                frame 10 {
                                }
                                frame 11 {
                                }
                                frame 12 {
                                }
                                frame 13 {
                                }
                                frame 14 {
                                }
                                frame 15 {
                                }
                                frame 16 {
                                }
                                frame 17 {
                                }
                                frame 18 {
                                }
                                frame 19 {
                                }
                                frame 20 {
                                }
                                }
                                n538 = Format Value(format string="%.3f", value (0)=w953) -> (output string=w957:string)  [unwired: 1 in]
                                n539 = call <vilib>:"Space Constant.vi"() -> ("String"=w958:string)
                                n540 = Concatenate Strings(w956, w955, w958, w957, w958) -> (w954:string)
                                }
                                frame True {
                                }
                                }
                              }
                              n541 = String Length(string=w936) -> (length=w937:i32)
                              n542 = Not Equal To 0?(x=w937) -> (x != 0?=w938:bool)
                              n543 = case shown="True" w938 {
                                tunnel: w946 -> [w981 w990]
                                tunnel: w945 -> [w982 w989]
                                tunnel: w936 -> [_ w985]
                                tunnel: [w981 w984] -> w899
                                tunnel: [w982 w983] -> w900
                                frame False {
                                }
                                frame True {
                                n544 = local read "IP_broadcast"() -> (w987:string)
                                n545 = local read "port_remote"() -> (w986:u16)
                                n546 = String To IP(1:w987) -> (0:w988:u32)
                                n547 = UDP Write(address=w988, port or service name=w986, connection ID=w990, data in=w985, 8:w989) -> (error out=w983:errorcluster, 3:w984:refnum<k16>)  [unwired: 1 in]
                                }
                              }
                              n548 = local read "VSmissed"() -> (w931:bool)
                              n549 = local read "stateMissed"() -> (w932:bool)
                              n550 = local read "CurTrial#"() -> (w928:u16)
                              n551 = local read "totalTrial#"() -> (w929:u16)
                              n552 = local read "run-stop"() -> (w935:bool)
                              n553 = Equal?(x=w928, y=w929) -> (x = y?=w930:bool)
                              n554 = Not(x=w935) -> (.not. x?=w934:bool)
                              n555 = Compound Arithmetic op=OR(w931, w932, w930) -> (w933:bool)
                              n556 = case shown="False" w933 {
                                frame False {
                                }
                                frame True {
                                n557 = local write "run-stop"(FALSE ("run-stop")) -> ()
                                }
                              }
                              n558 = Compound Arithmetic op=OR(w933, w934, w901) -> (w927:bool)
                            }
                            frame #1 {
                              n559 = UDP Read(connection ID=w997, timeout ms (25000)=0, 8:w996) -> (data out=w1000:string, error out=w1005:errorcluster, 3:w995:refnum<k16>, 6:w1001:u32)  [unwired: 1 in, 1 out]
                              n560 = String Length(string=w1000) -> (length=w1003:i32)
                              n561 = local write "Incoming data"(w1000) -> ()
                              n562 = Not Equal To 0?(x=w1003) -> (x != 0?=w1002:bool)
                              n563 = case shown="True" w1002 {
                                tunnel: w1001 -> [_ w1013]
                                tunnel: w1000 -> [_ w1019]
                                tunnel: w999 -> [w1007 w1012]
                                tunnel: [w1007 w1010] -> w998
                                tunnel: w992 -> [w1006 w1009]
                                tunnel: [w1006 w1008] -> w991
                                frame False {
                                }
                                frame True {
                                n564 = Scan From String(format string="%s %f ", input string=w1019, initial scan location=u32 0, default 1="no" ("default value 1"), default 2=-1.0 ("default value 2")) -> (output 1=w1014:string, output 2=w1011:dbl)  [unwired: 1 in, 3 out]
                                n565 = case shown="\"TrlDone\", Default" w1014 {
                                tunnel: w1013 -> [w1029]
                                tunnel: w1012 -> [w1022]
                                tunnel: w1011 -> [w1023]
                                tunnel: [w1022] -> w1010
                                tunnel: w1009 -> [w1021]
                                tunnel: [w1020] -> w1008
                                frame "TrlDone", Default {
                                n566 = local read "IP_RT"() -> (w1027:string)
                                n567 = IP To String(1:TRUE ("dot notation? (F)"), 2:w1029) -> (0:w1024:string)
                                n568 = Match True/False String(2:"" ("false string"), 3:w1027, 4:w1024) -> (0:w1025:bool)  [unwired: 1 out]
                                n569 = local write "Originating IP"(w1024) -> ()
                                n570 = case shown="True" w1025 {
                                tunnel: w1024 -> [w1036 _]
                                tunnel: w1022 -> [w1033 w1054]
                                tunnel: w1023 -> [w1032 w1048]
                                tunnel: w1021 -> [w1030 w1053]
                                tunnel: [w1030 w1052] -> w1020
                                frame False {
                                n571 = local read "IP_VS"() -> (w1035:string)
                                n572 = Match True/False String(2:"" ("false string"), 3:w1035, 4:w1036) -> (0:w1031:bool)  [unwired: 1 out]
                                n573 = case shown="True" w1031 {
                                tunnel: w1033 -> [_ w1043]
                                tunnel: w1032 -> [_ w1042]
                                frame False {
                                n574 = local write "Error 2"("Unknown source Error") -> ()
                                }
                                frame True {
                                n575 = Subtract(x=w1042, y=w1043) -> (x-y=w1041:dbl)
                                n576 = Absolute Value(x=w1041) -> (abs(x)=w1040:dbl)
                                n577 = local write "VSbusy"(FALSE) -> ()
                                n578 = Greater?(x=w1040, y=1e-06) -> (0:w1038:bool)
                                n579 = local write "VSmissed"(w1038) -> ()
                                }
                                }
                                }
                                frame True {
                                n580 = To Word Integer(number=w1048) -> (16bit integer=w1051:i16)
                                n581 = local read "forceCorrTrial"() -> (w1050:bool)
                                n582 = To Word Integer(number=w1048) -> (16bit integer=w1047:i16)
                                n583 = disable-structure shown="Disabled" {
                                disable-tunnel: w1048 -> [w1086 _]
                                disable-tunnel: w1054 -> [w1085 _]
                                frame Disabled {
                                n584 = Subtract(x=w1086, y=w1085) -> (x-y=w1084:dbl)
                                n585 = Absolute Value(x=w1084) -> (abs(x)=w1083:dbl)
                                n586 = Greater?(x=w1083, y=1e-06) -> (0:w1081:bool)
                                n587 = local write "stateMissed"(w1081) -> ()
                                }
                                frame Enabled {
                                }
                                }
                                n588 = local write "stateBusy"(FALSE) -> ()
                                n589 = case shown="0, Default" w1047 {
                                tunnel: [w1058 0] -> w1049
                                tunnel: [0 w1068] -> w1046
                                tunnel: [w1056 w1060] -> w1045
                                frame 0, Default {
                                n590 = local read "contNoRewardAccum"() -> (w1056:i32)
                                n591 = local read "contNoReward"() -> (w1059:i32)
                                n592 = Increment(x=w1059) -> (x+1=w1058:i32)
                                }
                                frame 1 {
                                n593 = local read "contNoReward"() -> (w1064:i32)
                                n594 = Greater?(x=w1064, y=5) -> (0:w1065:bool)
                                n595 = Select(t=w1064, s=w1065, f=0) -> (s? t:f=w1063:i32)
                                n596 = local read "contNoRewardAccum"() -> (w1062:i32)
                                n597 = local read "contReward"() -> (w1067:i32)
                                n598 = Add(x=w1063, y=w1062) -> (x+y=w1060:i32)
                                n599 = Increment(x=w1067) -> (x+1=w1068:i32)
                                }
                                }
                                n600 = case shown="True" w1050 {
                                tunnel: w1054 -> [_ w1074]
                                tunnel: w1053 -> [w1070 w1073]
                                tunnel: [w1070 w1072] -> w1052
                                tunnel: w1051 -> [_ w1071]
                                frame False {
                                }
                                frame True {
                                n601 = case shown="0" w1071 {
                                tunnel: w1074 -> [w1076 _]
                                tunnel: w1073 -> [w1079 w1080]
                                tunnel: [w1077 w1080] -> w1072
                                frame 0 {
                                n602 = Decrement(x=w1076) -> (x-1=w1075:i32)
                                n603 = Index Array(array=w1079, index=w1075) -> (element=w1078:i32)
                                n604 = Replace Array Subset(array=w1079, new element=w1078, index=w1076) -> (w1077:i32[])
                                }
                                frame 1, Default {
                                }
                                }
                                }
                                }
                                n605 = local write "contNoReward"(w1049) -> ()
                                n606 = local write "contReward"(w1046) -> ()
                                n607 = local write "contNoRewardAccum"(w1045) -> ()
                                }
                                }
                                }
                                }
                                }
                              }
                              n608 = call "Remove_selected_error.vi"("error in (no error)"=w1005, "errorCode"=56) -> ("error out"=w994:errorcluster)
                            }
                          }
                        }
                      }
                      n609 = local read "stop - local"() -> (w594:bool)
                      n610 = node-c288() -> ()  [unwired: 1 in, 1 out]
                    }
                    n611 = node-c288(w320) -> ()  [unwired: 1 out]
                    n612 = Release Queue(queue=w319, error in (no error)=w318) -> (error out=w308:errorcluster)  [unwired: 1 in, 2 out]
                    n613 = To Single Precision Float(number=w333) -> (single precision float=w335:sgl[][])
                    n614 = local read "Save data"() -> (w334:bool)
                    n615 = node-c288(w353) -> ()  [unwired: 1 out]
                    n616 = case shown="True" w334 {
                      tunnel: w314 -> [w568 w582]
                      tunnel: w315 -> [_ w581]
                      tunnel: w335 -> [_ w572]
                      tunnel: [w568 w569] -> w307
                      frame False {
                      }
                      frame True {
                        n617 = Multiply(x=502, y=4) -> (x*y=w577:i32)
                        n618 = Set File Position(offset (in bytes) (0)=w577, refnum=w581, from (0:start)=enum16{"start", "end", "current"}."start", error in=w582) -> (refnum out=w574:refnum<file>, error out=w575:errorcluster)
                        n619 = Write to Binary File(file (use dialog)=w574, data=w572, error in=w575, 5:FALSE ("prepend array or string size? (T)"), 9:T3."little-endian" ("byte order (0:big-endian, network order)")) -> (refnum out=w570:refnum<file>, error out=w571:errorcluster)  [unwired: 1 in, 1 out]
                        n620 = Close File(refnum=w570, error in=w571) -> (error out=w569:errorcluster)  [unwired: 1 out]
                      }
                    }
                    n621 = node-c288(w322) -> ()  [unwired: 1 out]
                    n622 = Release Queue(queue=w313, error in (no error)=w312) -> (error out=w287:errorcluster)  [unwired: 1 in, 2 out]
                    n623 = Destroy Stream Endpoint(8:w346, 11:w349) -> (0:w310:errorcluster)
                    n624 = node-c288(w344) -> ()  [unwired: 1 out]
                    n625 = flat-sequence {
                      tunnel: w305 -> [w392]
                      frame #0 {
                        n626 = call <vilib>:"Simple Error Handler.vi"("error in (no error)"=w392) -> ()  [unwired: 4 in, 5 out]
                        n627 = shared-variable "Sabrina-RT1\\variables - network - RT (separate).lvlib\\stop - network"(FALSE ("stop - network")) -> ()  [unwired: 1 in, 1 out]
                      }
                    }
                    n628 = UDP Close(connection ID=w283, 8:w282) -> ()  [unwired: 2 out]
                    n629 = UDP Close(connection ID=w340, 8:w339) -> (error out=w311:errorcluster)  [unwired: 1 out]
                    n630 = Merge Errors(w311, w310, w306, w309, w287, w308, w307) -> (w305:errorcluster)
                  }
                }
              }
              frame 2 {
                n631 = local read "IP_host"() -> (w1157:string)
                n632 = local read "port_local"() -> (w1158:u16)
                n633 = String To IP(1:w1157) -> (0:w1156:u32)
                n634 = UDP Open(7:w1156, 11:w1158) -> (port=w1160:refnum<k16>, 0:w1161:errorcluster)  [unwired: 3 in, 1 out]
                n635 = local read "IP_broadcast"() -> (w1154:string)
                n636 = local read "port_remote"() -> (w1155:u16)
                n637 = String To IP(1:w1154) -> (0:w1159:u32)
                n638 = UDP Write(address=w1159, port or service name=w1155, connection ID=w1160, data in="exit 1.000 ", 8:w1161) -> (error out=w1163:errorcluster, 3:w1162:refnum<k16>)  [unwired: 1 in]
                n639 = UDP Close(connection ID=w1162, 8:w1163) -> (error out=w1164:errorcluster)  [unwired: 1 out]
                n640 = call <vilib>:"Simple Error Handler.vi"("error in (no error)"=w1164) -> ()  [unwired: 4 in, 5 out]
              }
            }
          }
          frame #2 {
            n641 = Wait (ms)(milliseconds to wait=u32 5) -> ()  [unwired: 1 out]
          }
        }
      }
    }
  }
